vi "utility_panel.vi"() -> ()   [LabVIEW 2012]
doc: "This VI is to serve as (1) an example of how one might incorporate the many features of the stepper motor control API into their own application and (2) allows the user to take control of their hardware for demonstration and or troubleshooting purposes. Tips and descriptions have been applied to each control on the interface. Click the HELP button to see more detailed descriptions of each control and their function.\n\nProduced By:\n\nChristopher Lemieux\nKod Integrations, LLC\n4835 Marianne Drive\nMount Airy, MD 21771\nhttp://www.kodintegrations.com\nemail: clemieux@kodintegrations.com\nphone: (240) 687-1288"
uses:
  utilities/getters/controls/status_states.ctl
  support/controls/utility_actions.ctl
  main_functions/commands.ctl
  support/controls/digital_output_items.ctl
  support/controls/polarity_item_group.ctl
  support/controls/polarity_items.ctl
  support/controls/errors_actions.ctl
panel:
  in  "help":bool
  out "Current State (display)":T1(ring)=enum."CONST"
  out "Current Position (display)":i32=100 min=1 max=5000
  out "date":string
  out "power_led":bool
  in  "on/off":bool
  out "dig_ins":T2
  out "status":T3=enum."CONST"
  in  "jog_to_pos":i32 caption="Jog To Value"
  in  "move_to":bool caption="Jog To..."
  in  "home_neg":bool caption="Home (-)"
  in  "home_pos":bool caption="Home (+)"
  in  "clear":bool caption="Clear Error Codes"
  in  "Tab Control":T4(tab)
  in  "move_mode":enum32{"Abs:", "Inc:"}(radio)
  in  "position_val_set":bool
  out "position_val_actual":i32=100 min=1 max=5000
  in  "position_val_desired":i32
  in  "zero":bool
  in  "demo_start":bool
  in  "pos_3":i32
  in  "pos_2":i32
  in  "pos_1":i32
  in  "accel_set":bool
  out "accel_act":i32=100 min=1 max=5000
  in  "accel":i32=100 min=10 max=1000
  in  "low_speed_set":bool
  in  "high_speed_set":bool
  out "low_speed_act":i32=100 min=100 max=490550
  out "high_speed_act":i32=1 min=1 max=400000
  in  "low_speed":i32=100 min=100 max=490550
  in  "high_speed":i32=50 min=1 max=400000 step=1
  in  "dig_outs":T5
  out "actual_amp":i32
  in  "polarities":T6
  in  "cgh_id":bool
  in  "new_id":string
  in  "run_amp_set":bool
  in  "idle_amp_set":bool
  out "running_amp_act":i32
  out "idle_amp_act":i32
  in  "running_amp":i32=50 min=50 max=2500
  in  "idle_amp":i32=50 min=50 max=2500 step=1
  out "response":string
  out "firmware_ver":string
  out "dev_id":string
  out "prod_id":string
  in  "terminate":bool
  in  "jog_neg":bool caption="Jog (-)"
  in  "jog_pos":bool caption="Jog (+)"
  in  "imm_stop":bool caption="Stop Immediately"
  in  "slow_stop":bool caption="Stop Slowly"
  in  "raw_cmd":string
  in  "write_cmd":bool
  out "error out":errorcluster
  in  "error in (no error)":errorcluster
  # "Firmware:"
  # "Prod ID:"
  # "Dev ID:"
  # "Digital Inputs"
  # "Current Position"
  # "Current State"
  # "Status:"
  # "Mode"
  # "Speed Settings (pps)"
  # "set"
  # "(actual)"
  # "High"
  # "Low"
  # "Acceleration (ms)"
  # "set"
  # "(actual)"
  # "Accel"
  # "Demonstration"
  # "Zero First?"
  # "Position (1)"
  # "Position (2)"
  # "Position (3)"
  # "Position (ticks)"
  # "set"
  # "(actual)"
  # "new"
  # "Current Settings (mA)"
  # "set"
  # "(actual)"
  # "Idle"
  # "Run"
  # "[actual at runtime]"
  # "Polarity Settings:"
  # "Device ID:"
  # "Digital Outputs:"
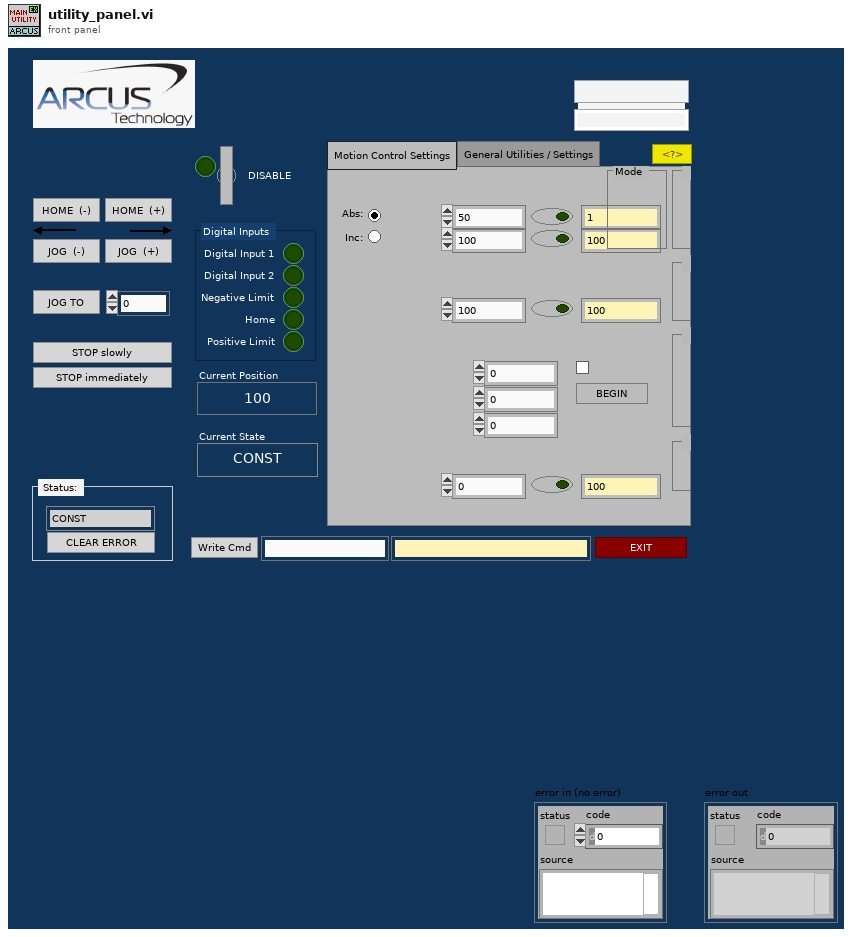
[diagram p1: front panel]
types:
  T1 = enum16{"IDLE", "CONST", "ACCEL", "DECEL", "HOME_SWITCH", "-LIMIT_SWITCH", "+LIMIT_SWITCH", "-LIMIT_ERR", "+LIMIT_ERR", "COMM_ERR"}
  T2 = cluster{"Digital Input 1":bool, "Digital Input 2":bool, "Negative Limit":bool, "Home":bool, "Positive Limit":bool}
  T3 = typedef "status_states.ctl" = enum16{"IDLE", "CONST", "ACCEL", "DECEL", "HOME_SWITCH", "-LIMIT_SWITCH", "+LIMIT_SWITCH", "-LIMIT_ERR", "+LIMIT_ERR", "COMM_ERR"}
  T4 = enum32{"Motion Control Settings", "General Utilities / Settings"}
  T5 = cluster{"Digital Output 1":bool, "Digital Output 2":bool}
  T6 = cluster{"Direction":bool, "Limit":bool, "Home":bool, "Digital Output":bool, "Digital Input":bool, "Enable Output":bool, "Jump On Error":bool}
  T7 = typedef "utility_actions.ctl" = enum16{"about", "clearError", "closeRef", "demo", "getAcceleration", "getActualCurrentVal", "getDeviceId", "getDeviceList", "getDigInputs", "getDigOutputs", "getDriverPowerStatus", "getFirmwareVer", "getHighSpeed", "getIdleCurrent", "getLowSpeed", "getMode", "getPolarity", "getPosition", "getProductId", "getRunCurrent", "getStatus", "homeMotorNeg", "homeMotorPos", "initialize", "jogConstNeg", "jogConstPos", "moveToPos", "openRef", "pause", "powerOFF", "powerON", "processEvents", "rawCmd", "setAcceleration", "setDeviceId", "setDigOutput", "setHighSpeed", "setLowSpeed", "setPolarity", "setPosition", "setRunCurrent", "setIdleCurrent", "setMode", "setTimeOuts", "stopImmediately", "stopSlowly", "storeToFlashMem", "updatePanelItems", "validateDemoPos", "validatePos", "waitUntilDone", "zeroPosition"}
  T8 = typedef "errors_actions.ctl" = enum16{"clearBuff", "closeRef", "noDeviceInfo", "noDevices", "openRef", "sendReceive", "setTimeouts", "unknown"}
  T9 = typedef "commands.ctl" = enum16{"clear error", "constant jog(-)", "constant jog(+)", "get acceleration", "get actual current", "get device id", "get digital input status", "get digial inputs status", "get dig output status", "get digital outputs status", "get firmware ver", "get high speed", "get idle current", "get low speed", "get micro step", "get motor status", "get move mode", "get polarity", "get position", "get product id", "get power status", "get run current", "get status", "home(-)", "home(+)", "move to position", "power down", "power up", "set acceleration", "set device id", "set digital output", "set digital outputs", "set high speed", "set idle current", "set low speed", "set move mode absolute", "set move mode increment", "set polarity", "set position", "set run current", "stop immediate", "stop slow", "store to memory"}
  T10 = typedef "digital_output_items.ctl" = enum16{"DIG_OUT_1", "DIG_OUT_2"}
  T11 = typedef "polarity_item_group.ctl" = cluster{"item":T12, "status":bool}
  T12 = typedef "polarity_items.ctl" = enum16{"DIRECTION", "LIMIT", "HOME", "DIG_OUT", "DIG_IN", "ENABLE_OUT", "JUMP_ERR"}
  T13 = cluster{"[0]":bool, "[1]":bool, "[2]":bool, "[3]":bool, "[4]":bool, "[5]":bool, "[6]":bool}
  T14 = typedef "digital_output_item_group.ctl" = cluster{"item":T10, "status":bool}
  T15 = typedef "digital_input_item_group.ctl" = cluster{"item":T16, "status":bool}
  T16 = typedef "digital_input_items.ctl" = enum16{"DIG_IN_1", "DIG_IN_2", "NEG_LIMIT", "HOME", "POS_LIMIT"}
  T17 = cluster{"[0]":bool, "[1]":bool, "[2]":bool, "[3]":bool, "[4]":bool}
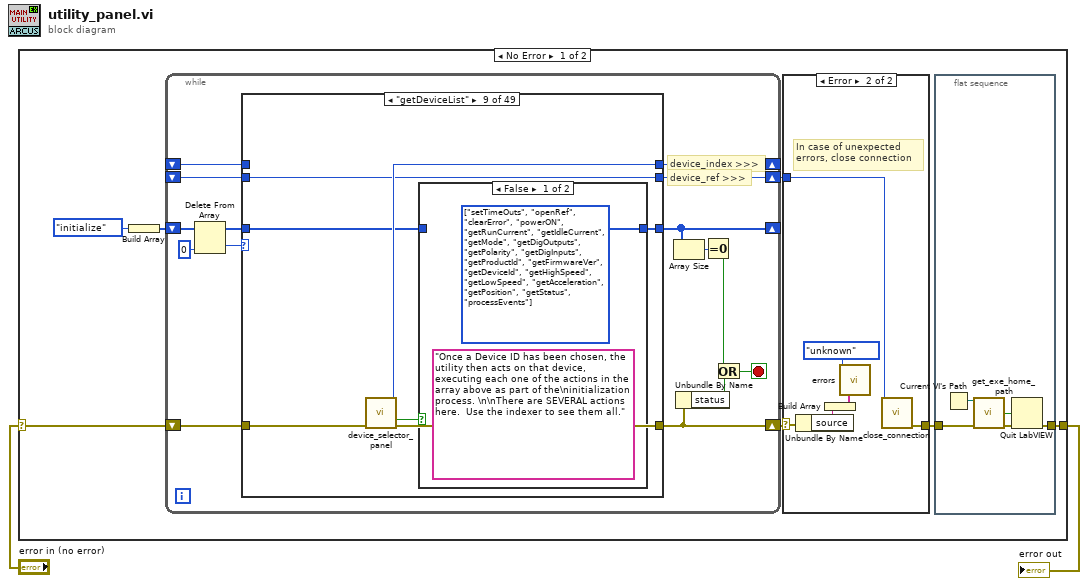
[diagram p0: block diagram]
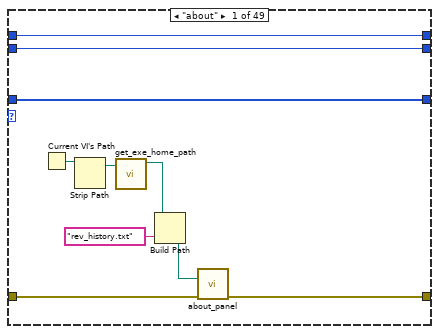
[diagram p3: hidden frame]
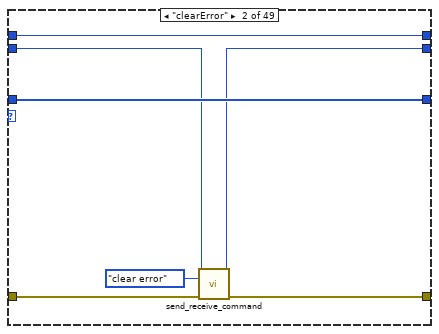
[diagram p4: hidden frame]
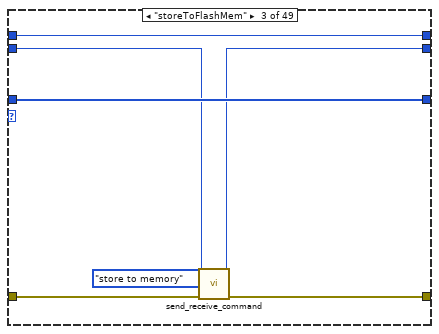
[diagram p5: hidden frame]
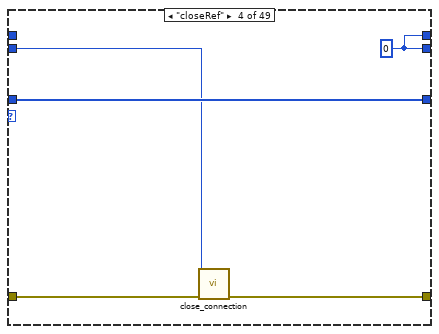
[diagram p6: hidden frame]
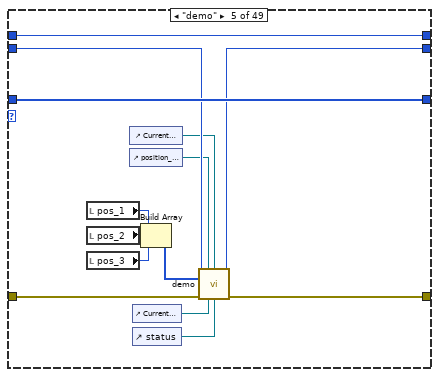
[diagram p7: hidden frame]
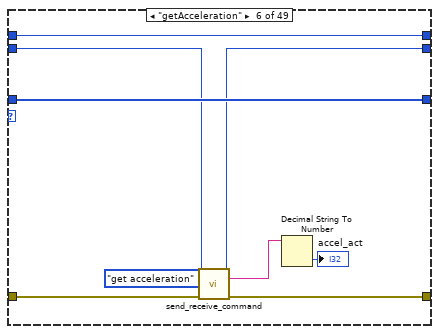
[diagram p8: hidden frame]
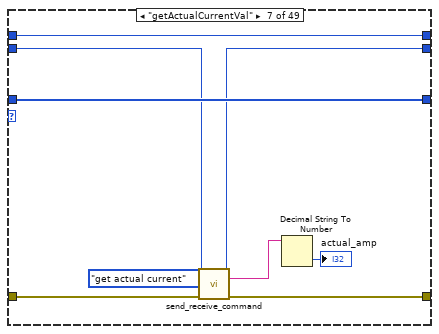
[diagram p9: hidden frame]
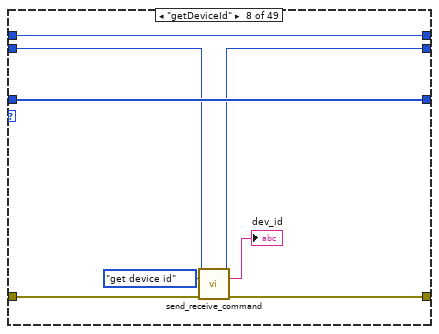
[diagram p10: hidden frame]
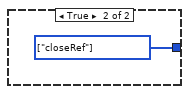
[diagram p11: hidden frame]
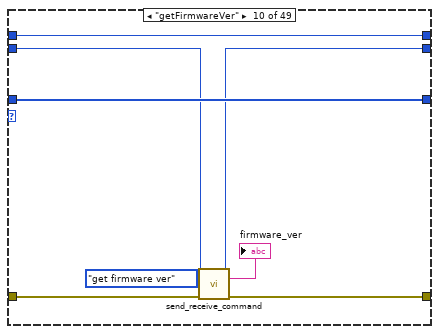
[diagram p12: hidden frame]
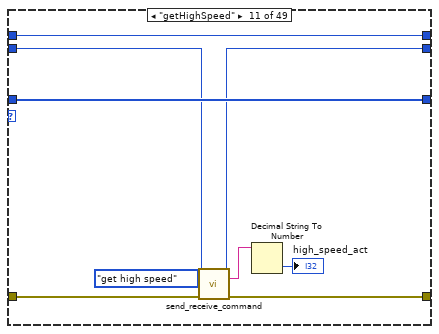
[diagram p13: hidden frame]
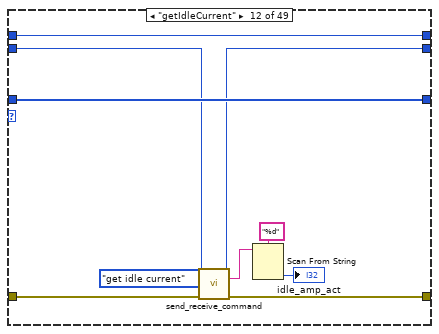
[diagram p14: hidden frame]
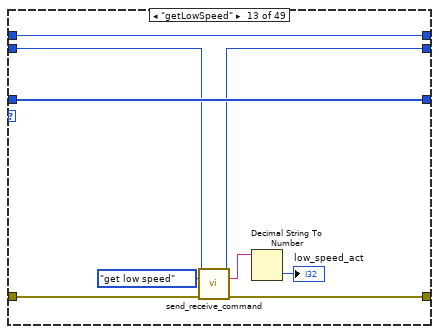
[diagram p15: hidden frame]
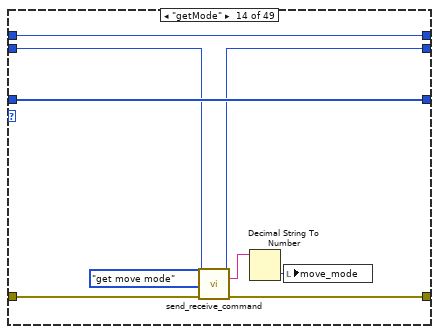
[diagram p16: hidden frame]
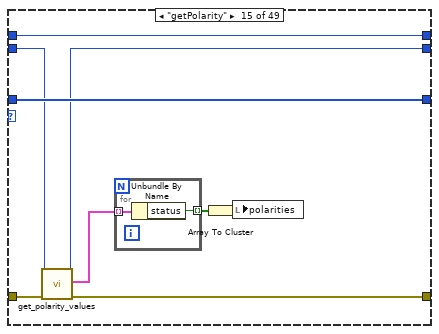
[diagram p17: hidden frame]
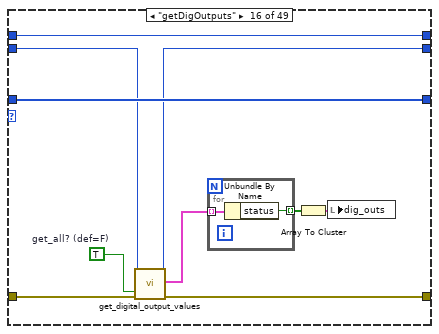
[diagram p18: hidden frame]
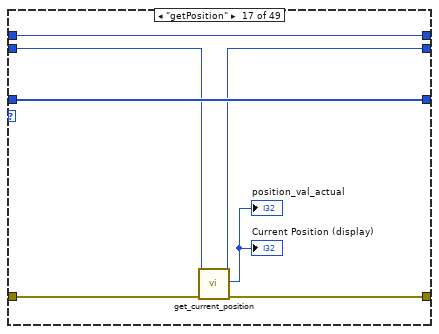
[diagram p19: hidden frame]
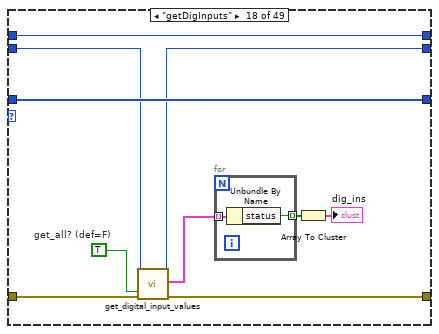
[diagram p20: hidden frame]
diagram:
  n1 = case shown="No Error" "error in (no error)" {
    selector: "error in (no error)" -> [w5 w614]
    tunnel: [w3 w614] -> w1
    frame No Error {
      n2 = Build Array(utility_actions."initialize" ("Enum")) -> (w8:T7[])
      n3 = while {
        shift-right: [w29] -> _
        shift-left: w8 -> [w34]
        shift-right: [w24] -> w7
        shift-left: w5 -> [w30]
        shift-right: [w23] -> w6
        shift-left: _ -> [w22]
        shift-right: [w21] -> _
        shift-left: _ -> [w20]
        stop <- w25 stop-if-true
        # "device_index >>>"
        # "device_ref >>>"
        n4 = Delete From Array(array=w34, index=0) -> (deleted portion=w32:T7, array with subset deleted=w31:T7[])  [unwired: 1 in]
        n5 = case shown="\"getDeviceList\"" w32 {
          tunnel: w31 -> [w44 w51 w58 w63 w73 w86 w95 w103 w105 w120 w129 w139 w148 w157 w166 w178 w187 w197 w207 w216 w223 w231 w239 _ w253 w261 w272 w278 w286 w294 w297 w399 w411 w424 w443 w455 w467 w477 w492 w502 w516 w528 w530 w544 w552 w556 w564 w590 w612]
          tunnel: [w44 w51 w58 w63 w73 w86 w95 w103 w104 w120 w129 w139 w148 w157 w166 w178 w187 w197 w207 w216 w223 w231 w239 w243 w253 w261 w271 w278 w286 w294 w298 w399 w410 w423 w442 w454 w466 w477 w491 w501 w515 w527 w530 w544 w552 w554 w560 w587 w611] -> w29
          tunnel: w30 -> [w41 w49 w56 w62 w72 w83 w93 w101 w110 w118 w127 w135 w146 w155 w164 w176 w185 w195 w205 w214 w221 w229 w237 w245 w251 w259 w270 w277 w283 w292 w301 w400 w408 w422 w440 w453 w465 w476 w490 w500 w514 w526 w534 w542 w550 w553 w561 w588 w610]
          tunnel: [w40 w48 w55 w61 w67 w82 w92 w100 w109 w117 w126 w134 w145 w154 w161 w173 w184 w194 w204 w213 w220 w225 w233 w245 w250 w258 w269 w276 w282 w291 w300 errorcluster {"status"=FALSE, "code"=0, "source"=""} w407 w414 w439 w452 w464 w475 w489 w499 w513 w525 w533 w541 w549 w553 w562 w589 w609] -> w24
          tunnel: [w42 w46 w53 w59 w70 w79 w89 w97 w107 w115 w124 w131 w143 w152 w162 w174 w182 w192 w202 w210 w218 w227 w235 w242 w248 w256 w267 w275 w280 w288 w295 w394 w405 w420 w434 w450 w462 w473 w487 w497 w511 w523 w535 w539 w547 w557 w578 w595 w607] -> w23
          tunnel: w22 -> [w42 w47 w54 w60 w71 w80 w90 w98 w107 w116 w125 w132 w144 w153 w163 w175 w183 w193 w203 w211 w219 w228 w236 _ w249 w257 w268 _ w281 w289 w295 w395 w406 w421 w438 w451 w463 w474 w488 w498 w512 w524 w535 w540 w548 w557 w578 w595 w608]
          tunnel: [w43 w50 w57 w59 w74 w85 w94 w102 w108 w119 w128 w138 w147 w156 w165 w177 w186 w196 w206 w215 w222 w230 w238 w242 w252 w260 w273 w274 w285 w293 w296 w396 w412 w425 w444 w456 w468 w478 w493 w503 w517 w529 w536 w543 w551 w558 w579 w596 w613] -> w21
          tunnel: w20 -> [w43 w50 w57 _ w74 w85 w94 w102 _ w119 w128 w138 w147 w156 w165 w177 w186 w196 w206 w215 w222 w230 w238 _ w252 w260 w273 w274 w285 w293 w296 w396 w412 w425 w444 w456 w468 w478 w493 w503 w517 w529 w536 w543 w551 w558 w579 w596 w613]
          frame "about" {
            n6 = Current VI's Path() -> (path=w37:path)
            n7 = Strip Path(path=w37) -> (stripped path=w36:path)  [unwired: 1 out]
            n8 = call "get_exe_home_path.vi"("home_path"=w36) -> ("actual_home_path"=w35:path)  [unwired: 6 in, 1 out]
            n9 = Build Path(base path=w35, name or relative path="rev_history.txt") -> (appended path=w38:path)
            n10 = call "about_panel.vi"("rev_history_filepath"=w38, "error in (no error)"=w41) -> ("error out"=w40:errorcluster)  [unwired: 13 in]
          }
          frame "clearError" {
            n11 = call "send_receive_command.vi"("reference (in)"=w47, "command"=commands."clear error" ("commands"), "error in (no error)"=w49) -> ("reference (dup)"=w46:i32, "error out"=w48:errorcluster)  [unwired: 8 in, 3 out]
          }
          frame "storeToFlashMem" {
            n12 = call "send_receive_command.vi"("reference (in)"=w54, "command"=commands."store to memory" ("commands"), "error in (no error)"=w56) -> ("reference (dup)"=w53:i32, "error out"=w55:errorcluster)  [unwired: 8 in, 3 out]
          }
          frame "closeRef" {
            w59 = 0 ("reference (out)")
            n13 = call "close_connection.vi"("reference"=w60, "error in (no error)"=w62) -> ("error out"=w61:errorcluster)  [unwired: 13 in]
          }
          frame "demo" {
            n14 = local read "pos_1"() -> (w76:i32)
            n15 = local read "pos_2"() -> (w75:i32)
            n16 = local read "pos_3"() -> (w77:i32)
            n17 = control-ref of="Current Position (display)"() -> (w66:refnum<vi>)
            n18 = control-ref of="position_val_actual"() -> (w69:refnum<vi>)
            n19 = control-ref of="Current State (display)"() -> (w65:refnum<vi>)
            n20 = control-ref of="status"() -> (w64:refnum<vi>)
            n21 = Build Array(w76, w75, w77) -> (w68:i32[])
            n22 = call "demo.vi"("reference (in)"=w71, "position ref"=w69, "position (large) ref"=w66, "positions"=w68, "error in (no error)"=w72, "Current State (display)"=w65, "status"=w64) -> ("reference (out)"=w70:i32, "error out"=w67:errorcluster)  [unwired: 7 in]
          }
          frame "getAcceleration" {
            n23 = call "send_receive_command.vi"("reference (in)"=w80, "command"=commands."get acceleration" ("commands"), "error in (no error)"=w83) -> ("reference (dup)"=w79:i32, "read_string"=w78:string, "error out"=w82:errorcluster)  [unwired: 8 in, 2 out]
            n24 = Decimal String To Number(string=w78) -> (number=→"accel_act":i32)  [unwired: 2 in, 1 out]
          }
          frame "getActualCurrentVal" {
            n25 = call "send_receive_command.vi"("reference (in)"=w90, "command"=commands."get actual current" ("commands"), "error in (no error)"=w93) -> ("reference (dup)"=w89:i32, "read_string"=w88:string, "error out"=w92:errorcluster)  [unwired: 8 in, 2 out]
            n26 = Decimal String To Number(string=w88) -> (number=→"actual_amp":i32)  [unwired: 2 in, 1 out]
          }
          frame "getDeviceId" {
            n27 = call "send_receive_command.vi"("reference (in)"=w98, "command"=commands."get device id" ("commands"), "error in (no error)"=w101) -> ("reference (dup)"=w97:i32, "read_string"=→"dev_id":string, "error out"=w100:errorcluster)  [unwired: 8 in, 2 out]
          }
          frame "getDeviceList" {
            n28 = call "device_selector_panel.vi"("error in (no error)"=w110) -> ("index"=w108:i32, "cancel?"=w106:bool, "error out"=w109:errorcluster)  [unwired: 10 in, 2 out]
            n29 = case shown="False" w106 {
              tunnel: w105 -> [_ _]
              tunnel: [w111 w112] -> w104
              frame False {
                (unwired) "Once a Device ID has been chosen, the utility then acts on that device, executing each one of the actions in the array above as part of the\ninitialization process. \n\nThere are SEVERAL actions here.  Use the indexer to see them all."
                w111 = T7[] [enum."setTimeOuts", enum."openRef", enum."clearError", enum."powerON", enum."getRunCurrent", enum."getIdleCurrent", enum."getMode", enum."getDigOutputs", enum."getPolarity", enum."getDigInputs", enum."getProductId", enum."getFirmwareVer", enum."getDeviceId", enum."getHighSpeed", enum."getLowSpeed", enum."getAcceleration", enum."getPosition", enum."getStatus", enum."processEvents"] items=["about", "clearError", "closeRef", "demo", "getAcceleration", "getActualCurrentVal", "getDeviceId", "getDeviceList", "getDigInputs", "getDigOutputs", "getDriverPowerStatus", "getFirmwareVer", "getHighSpeed", "getIdleCurrent", "getLowSpeed", "getMode", "getPolarity", "getPosition", "getProductId", "getRunCurrent", "getStatus", "homeMotorNeg", "homeMotorPos", "initialize", "jogConstNeg", "jogConstPos", "moveToPos", "openRef", "pause", "powerOFF", "powerON", "processEvents", "rawCmd", "setAcceleration", "setDeviceId", "setDigOutput", "setHighSpeed", "setLowSpeed", "setPolarity", "setPosition", "setRunCurrent", "setIdleCurrent", "setMode", "setTimeOuts", "stopImmediately", "stopSlowly", "storeToFlashMem", "updatePanelItems", "validateDemoPos", "validatePos", "waitUntilDone", "zeroPosition"] ("actions")
              }
              frame True {
                w112 = T7[] [enum."closeRef"] items=["about", "clearError", "closeRef", "demo", "getAcceleration", "getActualCurrentVal", "getDeviceId", "getDeviceList", "getDigInputs", "getDigOutputs", "getDriverPowerStatus", "getFirmwareVer", "getHighSpeed", "getIdleCurrent", "getLowSpeed", "getMode", "getPolarity", "getPosition", "getProductId", "getRunCurrent", "getStatus", "homeMotorNeg", "homeMotorPos", "initialize", "jogConstNeg", "jogConstPos", "moveToPos", "openRef", "pause", "powerOFF", "powerON", "processEvents", "rawCmd", "setAcceleration", "setDeviceId", "setDigOutput", "setHighSpeed", "setLowSpeed", "setPolarity", "setPosition", "setRunCurrent", "setIdleCurrent", "setMode", "setTimeOuts", "stopImmediately", "stopSlowly", "storeToFlashMem", "updatePanelItems", "validateDemoPos", "validatePos", "waitUntilDone", "zeroPosition"] ("actions")
              }
            }
          }
          frame "getFirmwareVer" {
            n30 = call "send_receive_command.vi"("reference (in)"=w116, "command"=commands."get firmware ver" ("commands"), "error in (no error)"=w118) -> ("reference (dup)"=w115:i32, "read_string"=→"firmware_ver":string, "error out"=w117:errorcluster)  [unwired: 8 in, 2 out]
          }
          frame "getHighSpeed" {
            n31 = call "send_receive_command.vi"("reference (in)"=w125, "command"=commands."get high speed" ("commands"), "error in (no error)"=w127) -> ("reference (dup)"=w124:i32, "read_string"=w121:string, "error out"=w126:errorcluster)  [unwired: 8 in, 2 out]
            n32 = Decimal String To Number(string=w121) -> (number=→"high_speed_act":i32)  [unwired: 2 in, 1 out]
          }
          frame "getIdleCurrent" {
            n33 = call "send_receive_command.vi"("reference (in)"=w132, "command"=commands."get idle current" ("commands"), "error in (no error)"=w135) -> ("reference (dup)"=w131:i32, "read_string"=w130:string, "error out"=w134:errorcluster)  [unwired: 8 in, 2 out]
            n34 = Scan From String(format string="%d", input string=w130) -> (output 1=→"idle_amp_act":i32)  [unwired: 3 in, 3 out]
          }
          frame "getLowSpeed" {
            n35 = call "send_receive_command.vi"("reference (in)"=w144, "command"=commands."get low speed" ("commands"), "error in (no error)"=w146) -> ("reference (dup)"=w143:i32, "read_string"=w140:string, "error out"=w145:errorcluster)  [unwired: 8 in, 2 out]
            n36 = Decimal String To Number(string=w140) -> (number=→"low_speed_act":i32)  [unwired: 2 in, 1 out]
          }
          frame "getMode" {
            n37 = call "send_receive_command.vi"("reference (in)"=w153, "command"=commands."get move mode" ("commands"), "error in (no error)"=w155) -> ("reference (dup)"=w152:i32, "read_string"=w150:string, "error out"=w154:errorcluster)  [unwired: 8 in, 2 out]
            n38 = Decimal String To Number(string=w150) -> (number=w149:i32)  [unwired: 2 in, 1 out]
            n39 = local write "move_mode"(w149) -> ()
          }
          frame "getPolarity" {
            n40 = call "get_polarity_values.vi"("reference (in)"=w163, "error in (no error)"=w164) -> ("reference (dup)"=w162:i32, "polarity_items"=w160:T11[], "error out"=w161:errorcluster)  [unwired: 14 in, 1 out]
            n41 = for {
              tunnel: w160 -> [w168] mode=indexing
              tunnel: [w167] -> w159 mode=indexing
              n42 = Unbundle By Name(w168) -> ("status"=w167:bool)
            }
            n43 = Array To Cluster(array=w159) -> (cluster=w158:T13)
            n44 = local write "polarities"(w158) -> ()
          }
          frame "getDigOutputs" {
            w169 = TRUE  # get_all? (def=F)
            n45 = call "get_digital_output_values.vi"("reference (in)"=w175, "get_all? (def=F)"=w169, "error in (no error)"=w176) -> ("reference (dup)"=w174:i32, "do_items"=w172:T14[], "error out"=w173:errorcluster)  [unwired: 12 in, 2 out]
            n46 = for {
              tunnel: w172 -> [w180] mode=indexing
              tunnel: [w179] -> w171 mode=indexing
              n47 = Unbundle By Name(w180) -> ("status"=w179:bool)
            }
            n48 = Array To Cluster(array=w171) -> (cluster=w170:cluster{"[0]":bool, "[1]":bool})
            n49 = local write "dig_outs"(w170) -> ()
          }
          frame "getPosition" {
            n50 = call "get_current_position.vi"("reference (in)"=w183, "error in (no error)"=w185) -> ("reference (dup)"=w182:i32, "current_position (units)"=→"position_val_actual" →"Current Position (display)":i32, "error out"=w184:errorcluster)  [unwired: 15 in]
          }
          frame "getDigInputs" {
            w188 = TRUE  # get_all? (def=F)
            n51 = call "get_digital_input_values.vi"("reference (in)"=w193, "get_all? (def=F)"=w188, "error in (no error)"=w195) -> ("reference (dup)"=w192:i32, "di_items"=w191:T15[], "error out"=w194:errorcluster)  [unwired: 12 in, 2 out]
            n52 = for {
              tunnel: w191 -> [w199] mode=indexing
              tunnel: [w198] -> w190 mode=indexing
              n53 = Unbundle By Name(w199) -> ("status"=w198:bool)
            }
            n54 = Array To Cluster(array=w190) -> (cluster=→"dig_ins":T17)
          }
          frame "getProductId" {
            n55 = call "send_receive_command.vi"("reference (in)"=w203, "command"=commands."get product id" ("commands"), "error in (no error)"=w205) -> ("reference (dup)"=w202:i32, "read_string"=→"prod_id":string, "error out"=w204:errorcluster)  [unwired: 8 in, 2 out]
          }
          frame "getRunCurrent" {
            n56 = call "send_receive_command.vi"("reference (in)"=w211, "command"=commands."get run current" ("commands"), "error in (no error)"=w214) -> ("reference (dup)"=w210:i32, "read_string"=w209:string, "error out"=w213:errorcluster)  [unwired: 8 in, 2 out]
            n57 = Decimal String To Number(string=w209) -> (number=→"running_amp_act":i32)  [unwired: 2 in, 1 out]
          }
          frame "getStatus" {
            n58 = call "get_status.vi"("reference (in)"=w219, "error in (no error)"=w221) -> ("reference (dup)"=w218:i32, "motion_state"=→"status" →"Current State (display)":T3, "error out"=w220:errorcluster)  [unwired: 13 in, 2 out]
          }
          frame "homeMotorNeg" {
            w224 = u8 2 ("Disabled")
            n59 = call "send_receive_command.vi"("reference (in)"=w228, "command"=commands."home(-)" ("commands"), "error in (no error)"=w229) -> ("reference (dup)"=w227:i32, "error out"=w225:errorcluster)  [unwired: 8 in, 3 out]
            n60 = property on="home_neg" class="Bool"("Disabled"=w224) -> ()  [unwired: 2 in, 2 out]
            n61 = property on="home_pos" class="Bool"("Disabled"=w224) -> ()  [unwired: 2 in, 2 out]
            n62 = property on="move_to" class="Bool"("Disabled"=w224) -> ()  [unwired: 2 in, 2 out]
            n63 = property on="jog_pos" class="Bool"("Disabled"=w224) -> ()  [unwired: 2 in, 2 out]
            n64 = property on="jog_neg" class="Bool"("Disabled"=w224) -> ()  [unwired: 2 in, 2 out]
          }
          frame "homeMotorPos" {
            w232 = u8 2 ("Disabled")
            n65 = call "send_receive_command.vi"("reference (in)"=w236, "command"=commands."home(+)" ("commands"), "error in (no error)"=w237) -> ("reference (dup)"=w235:i32, "error out"=w233:errorcluster)  [unwired: 8 in, 3 out]
            n66 = property on="home_neg" class="Bool"("Disabled"=w232) -> ()  [unwired: 2 in, 2 out]
            n67 = property on="home_pos" class="Bool"("Disabled"=w232) -> ()  [unwired: 2 in, 2 out]
            n68 = property on="move_to" class="Bool"("Disabled"=w232) -> ()  [unwired: 2 in, 2 out]
            n69 = property on="jog_pos" class="Bool"("Disabled"=w232) -> ()  [unwired: 2 in, 2 out]
            n70 = property on="jog_neg" class="Bool"("Disabled"=w232) -> ()  [unwired: 2 in, 2 out]
          }
          frame "initialize", Default {
            w240 = u8 0 ("Disabled")
            w243 = T7[] [enum."getDeviceList"] items=["about", "clearError", "closeRef", "demo", "getAcceleration", "getActualCurrentVal", "getDeviceId", "getDeviceList", "getDigInputs", "getDigOutputs", "getDriverPowerStatus", "getFirmwareVer", "getHighSpeed", "getIdleCurrent", "getLowSpeed", "getMode", "getPolarity", "getPosition", "getProductId", "getRunCurrent", "getStatus", "homeMotorNeg", "homeMotorPos", "initialize", "jogConstNeg", "jogConstPos", "moveToPos", "openRef", "pause", "powerOFF", "powerON", "processEvents", "rawCmd", "setAcceleration", "setDeviceId", "setDigOutput", "setHighSpeed", "setLowSpeed", "setPolarity", "setPosition", "setRunCurrent", "setIdleCurrent", "setMode", "setTimeOuts", "stopImmediately", "stopSlowly", "storeToFlashMem", "updatePanelItems", "validateDemoPos", "validatePos", "waitUntilDone", "zeroPosition"] ("actions")
            w242 = 0 ("index")
            w241 = ""
            w244 = FALSE
            n71 = local write "raw_cmd"(w241) -> ()
            n72 = local write "on/off"(w244) -> ()
            n73 = local write "power_led"(w244) -> ()
            n74 = local write "new_id"(w241) -> ()
            n75 = local write "response"(w241) -> ()
            n76 = property on="home_neg" class="Bool"("Disabled"=w240) -> ()  [unwired: 2 in, 2 out]
            n77 = property on="home_pos" class="Bool"("Disabled"=w240) -> ()  [unwired: 2 in, 2 out]
            n78 = property on="move_to" class="Bool"("Disabled"=w240) -> ()  [unwired: 2 in, 2 out]
            n79 = property on="jog_pos" class="Bool"("Disabled"=w240) -> ()  [unwired: 2 in, 2 out]
            n80 = property on="jog_neg" class="Bool"("Disabled"=w240) -> ()  [unwired: 2 in, 2 out]
          }
          frame "jogConstNeg" {
            w246 = u8 2 ("Disabled")
            n81 = call "send_receive_command.vi"("reference (in)"=w249, "command"=commands."constant jog(-)" ("commands"), "error in (no error)"=w251) -> ("reference (dup)"=w248:i32, "error out"=w250:errorcluster)  [unwired: 8 in, 3 out]
            n82 = property on="home_neg" class="Bool"("Disabled"=w246) -> ()  [unwired: 2 in, 2 out]
            n83 = property on="home_pos" class="Bool"("Disabled"=w246) -> ()  [unwired: 2 in, 2 out]
            n84 = property on="move_to" class="Bool"("Disabled"=w246) -> ()  [unwired: 2 in, 2 out]
            n85 = property on="jog_pos" class="Bool"("Disabled"=w246) -> ()  [unwired: 2 in, 2 out]
            n86 = property on="jog_neg" class="Bool"("Disabled"=w246) -> ()  [unwired: 2 in, 2 out]
          }
          frame "jogConstPos" {
            w254 = u8 2 ("Disabled")
            n87 = call "send_receive_command.vi"("reference (in)"=w257, "command"=commands."constant jog(+)" ("commands"), "error in (no error)"=w259) -> ("reference (dup)"=w256:i32, "error out"=w258:errorcluster)  [unwired: 8 in, 3 out]
            n88 = property on="home_neg" class="Bool"("Disabled"=w254) -> ()  [unwired: 2 in, 2 out]
            n89 = property on="home_pos" class="Bool"("Disabled"=w254) -> ()  [unwired: 2 in, 2 out]
            n90 = property on="move_to" class="Bool"("Disabled"=w254) -> ()  [unwired: 2 in, 2 out]
            n91 = property on="jog_pos" class="Bool"("Disabled"=w254) -> ()  [unwired: 2 in, 2 out]
            n92 = property on="jog_neg" class="Bool"("Disabled"=w254) -> ()  [unwired: 2 in, 2 out]
          }
          frame "moveToPos" {
            n93 = local read "jog_to_pos"() -> (w264:i32)
            n94 = Number To Decimal String(number=w264) -> (decimal integer string=w263:string)  [unwired: 1 in]
            n95 = Build Array(w263) -> (w266:string[])
            n96 = call "send_receive_command.vi"("reference (in)"=w268, "command"=commands."move to position" ("commands"), "params (opt)"=w266, "error in (no error)"=w270) -> ("reference (dup)"=w267:i32, "error out"=w269:errorcluster)  [unwired: 7 in, 3 out]
            n97 = Build Array (concatenate)(utility_actions."getPosition" ("Enum"), w272) -> (w271:T7[])
          }
          frame "openRef" {
            n98 = call "create_connection.vi"("device_index (def=0)"=w274, "error in (no error)"=w277) -> ("reference"=w275:i32, "error out"=w276:errorcluster)  [unwired: 12 in]
          }
          frame "powerOFF" {
            w279 = FALSE
            w284 = FALSE  # state (def=OFF)
            # "in the event this \ncase is triggered by\nsomething other \nthan the toggle"
            n99 = call "set_enable_disable_state.vi"("reference (in)"=w281, "state (def=OFF)"=w284, "error in (no error)"=w283) -> ("reference (dup)"=w280:i32, "error out"=w282:errorcluster)  [unwired: 14 in, 1 out]
            n100 = local write "power_led"(w279) -> ()
            n101 = local write "on/off"(w279) -> ()
          }
          frame "powerON" {
            w287 = TRUE
            w290 = TRUE  # state (def=OFF)
            # "in the event this \ncase is triggered by\nsomething other \nthan the toggle"
            n102 = call "set_enable_disable_state.vi"("reference (in)"=w289, "state (def=OFF)"=w290, "error in (no error)"=w292) -> ("reference (dup)"=w288:i32, "error out"=w291:errorcluster)  [unwired: 14 in, 1 out]
            n103 = local write "power_led"(w287) -> ()
            n104 = local write "on/off"(w287) -> ()
          }
          frame "processEvents" {
            n105 = event shown="[10] \"cgh_id\": Value Change" {
              selector: _ -> [_ _ _ _ _ _ _ _ _ _ _ _ _ _ _ _ _ _ _ _ _ _ _ _ _]
              dyn-events: _ -> [_ _ _ _ _ _ _ _ _ _ _ _ _ _ _ _ _ _ _ _ _ _ _ _ _]
              timeout: 20 -> [_ _ _ _ _ _ _ _ _ _ _ _ _ _ _ _ _ _ _ _ _ _ _ _ _]
              tunnel: [w305 w307 w309 w311 w313 w315 w317 w320 w324 w326 w335 w339 w341 w343 w345 w347 w349 w351 w354 w358 w359 w384 w388 w390 w392] -> w300
              tunnel: w301 -> [w305 w307 w309 w311 w313 w315 w317 w320 w324 w326 w335 w339 w341 w343 w345 w347 w349 w351 w354 w358 w359 w384 w388 w390 w392]
              tunnel: [w304 w306 w308 w310 w312 w314 w316 w319 w323 w325 w334 w338 w340 w342 w344 w346 w348 w350 w353 w357 w360 w383 w387 w389 w391] -> w298
              tunnel: w297 -> [_ _ _ _ _ _ _ _ _ _ _ _ _ _ _ _ _ _ _ _ _ _ _ _ _]
              event Timeout {
                w304 = T7[] [enum."updatePanelItems", enum."getDigInputs", enum."getPosition", enum."getStatus", enum."getActualCurrentVal", enum."processEvents"] items=["about", "clearError", "closeRef", "demo", "getAcceleration", "getActualCurrentVal", "getDeviceId", "getDeviceList", "getDigInputs", "getDigOutputs", "getDriverPowerStatus", "getFirmwareVer", "getHighSpeed", "getIdleCurrent", "getLowSpeed", "getMode", "getPolarity", "getPosition", "getProductId", "getRunCurrent", "getStatus", "homeMotorNeg", "homeMotorPos", "initialize", "jogConstNeg", "jogConstPos", "moveToPos", "openRef", "pause", "powerOFF", "powerON", "processEvents", "rawCmd", "setAcceleration", "setDeviceId", "setDigOutput", "setHighSpeed", "setLowSpeed", "setPolarity", "setPosition", "setRunCurrent", "setIdleCurrent", "setMode", "setTimeOuts", "stopImmediately", "stopSlowly", "storeToFlashMem", "updatePanelItems", "validateDemoPos", "validatePos", "waitUntilDone", "zeroPosition"] ("actions")
                n106 = event-data() -> ()  [unwired: 1 in, 2 out]
                n107 = Format Date/Time String(time format string (%c)="%B %d, %Y - %H:%M:%S") -> (date/time string=→"date":string)  [unwired: 2 in]
              }
              event "write_cmd": Value Change {
                w306 = T7[] [enum."rawCmd", enum."processEvents"] items=["about", "clearError", "closeRef", "demo", "getAcceleration", "getActualCurrentVal", "getDeviceId", "getDeviceList", "getDigInputs", "getDigOutputs", "getDriverPowerStatus", "getFirmwareVer", "getHighSpeed", "getIdleCurrent", "getLowSpeed", "getMode", "getPolarity", "getPosition", "getProductId", "getRunCurrent", "getStatus", "homeMotorNeg", "homeMotorPos", "initialize", "jogConstNeg", "jogConstPos", "moveToPos", "openRef", "pause", "powerOFF", "powerON", "processEvents", "rawCmd", "setAcceleration", "setDeviceId", "setDigOutput", "setHighSpeed", "setLowSpeed", "setPolarity", "setPosition", "setRunCurrent", "setIdleCurrent", "setMode", "setTimeOuts", "stopImmediately", "stopSlowly", "storeToFlashMem", "updatePanelItems", "validateDemoPos", "validatePos", "waitUntilDone", "zeroPosition"] ("actions")
                n108 = event-data() -> ()  [unwired: 1 in, 6 out]
              }
              event "slow_stop": Value Change {
                w308 = T7[] [enum."stopSlowly", enum."processEvents"] items=["about", "clearError", "closeRef", "demo", "getAcceleration", "getActualCurrentVal", "getDeviceId", "getDeviceList", "getDigInputs", "getDigOutputs", "getDriverPowerStatus", "getFirmwareVer", "getHighSpeed", "getIdleCurrent", "getLowSpeed", "getMode", "getPolarity", "getPosition", "getProductId", "getRunCurrent", "getStatus", "homeMotorNeg", "homeMotorPos", "initialize", "jogConstNeg", "jogConstPos", "moveToPos", "openRef", "pause", "powerOFF", "powerON", "processEvents", "rawCmd", "setAcceleration", "setDeviceId", "setDigOutput", "setHighSpeed", "setLowSpeed", "setPolarity", "setPosition", "setRunCurrent", "setIdleCurrent", "setMode", "setTimeOuts", "stopImmediately", "stopSlowly", "storeToFlashMem", "updatePanelItems", "validateDemoPos", "validatePos", "waitUntilDone", "zeroPosition"] ("actions")
                n109 = event-data() -> ()  [unwired: 1 in, 6 out]
              }
              event "imm_stop": Value Change {
                w310 = T7[] [enum."stopImmediately", enum."processEvents"] items=["about", "clearError", "closeRef", "demo", "getAcceleration", "getActualCurrentVal", "getDeviceId", "getDeviceList", "getDigInputs", "getDigOutputs", "getDriverPowerStatus", "getFirmwareVer", "getHighSpeed", "getIdleCurrent", "getLowSpeed", "getMode", "getPolarity", "getPosition", "getProductId", "getRunCurrent", "getStatus", "homeMotorNeg", "homeMotorPos", "initialize", "jogConstNeg", "jogConstPos", "moveToPos", "openRef", "pause", "powerOFF", "powerON", "processEvents", "rawCmd", "setAcceleration", "setDeviceId", "setDigOutput", "setHighSpeed", "setLowSpeed", "setPolarity", "setPosition", "setRunCurrent", "setIdleCurrent", "setMode", "setTimeOuts", "stopImmediately", "stopSlowly", "storeToFlashMem", "updatePanelItems", "validateDemoPos", "validatePos", "waitUntilDone", "zeroPosition"] ("actions")
                n110 = event-data() -> ()  [unwired: 1 in, 6 out]
              }
              event "jog_pos": Value Change {
                w312 = T7[] [enum."jogConstPos", enum."processEvents"] items=["about", "clearError", "closeRef", "demo", "getAcceleration", "getActualCurrentVal", "getDeviceId", "getDeviceList", "getDigInputs", "getDigOutputs", "getDriverPowerStatus", "getFirmwareVer", "getHighSpeed", "getIdleCurrent", "getLowSpeed", "getMode", "getPolarity", "getPosition", "getProductId", "getRunCurrent", "getStatus", "homeMotorNeg", "homeMotorPos", "initialize", "jogConstNeg", "jogConstPos", "moveToPos", "openRef", "pause", "powerOFF", "powerON", "processEvents", "rawCmd", "setAcceleration", "setDeviceId", "setDigOutput", "setHighSpeed", "setLowSpeed", "setPolarity", "setPosition", "setRunCurrent", "setIdleCurrent", "setMode", "setTimeOuts", "stopImmediately", "stopSlowly", "storeToFlashMem", "updatePanelItems", "validateDemoPos", "validatePos", "waitUntilDone", "zeroPosition"] ("actions")
                n111 = event-data() -> ()  [unwired: 1 in, 6 out]
              }
              event "jog_neg": Value Change {
                w314 = T7[] [enum."jogConstNeg", enum."processEvents"] items=["about", "clearError", "closeRef", "demo", "getAcceleration", "getActualCurrentVal", "getDeviceId", "getDeviceList", "getDigInputs", "getDigOutputs", "getDriverPowerStatus", "getFirmwareVer", "getHighSpeed", "getIdleCurrent", "getLowSpeed", "getMode", "getPolarity", "getPosition", "getProductId", "getRunCurrent", "getStatus", "homeMotorNeg", "homeMotorPos", "initialize", "jogConstNeg", "jogConstPos", "moveToPos", "openRef", "pause", "powerOFF", "powerON", "processEvents", "rawCmd", "setAcceleration", "setDeviceId", "setDigOutput", "setHighSpeed", "setLowSpeed", "setPolarity", "setPosition", "setRunCurrent", "setIdleCurrent", "setMode", "setTimeOuts", "stopImmediately", "stopSlowly", "storeToFlashMem", "updatePanelItems", "validateDemoPos", "validatePos", "waitUntilDone", "zeroPosition"] ("actions")
                n112 = event-data() -> ()  [unwired: 1 in, 6 out]
              }
              event "terminate": Value Change {
                w316 = T7[] [enum."powerOFF", enum."closeRef"] items=["about", "clearError", "closeRef", "demo", "getAcceleration", "getActualCurrentVal", "getDeviceId", "getDeviceList", "getDigInputs", "getDigOutputs", "getDriverPowerStatus", "getFirmwareVer", "getHighSpeed", "getIdleCurrent", "getLowSpeed", "getMode", "getPolarity", "getPosition", "getProductId", "getRunCurrent", "getStatus", "homeMotorNeg", "homeMotorPos", "initialize", "jogConstNeg", "jogConstPos", "moveToPos", "openRef", "pause", "powerOFF", "powerON", "processEvents", "rawCmd", "setAcceleration", "setDeviceId", "setDigOutput", "setHighSpeed", "setLowSpeed", "setPolarity", "setPosition", "setRunCurrent", "setIdleCurrent", "setMode", "setTimeOuts", "stopImmediately", "stopSlowly", "storeToFlashMem", "updatePanelItems", "validateDemoPos", "validatePos", "waitUntilDone", "zeroPosition"] ("actions")
                n113 = event-data() -> ()  [unwired: 1 in, 6 out]
              }
              event "on/off": Value Change {
                n114 = event-data() -> ("NewVal"=w318:bool)  [unwired: 1 in, 5 out]
                "power_led" <- w318
                n115 = case shown="False" w318 {
                  tunnel: [w321 w322] -> w319
                  frame True {
                    w321 = T7[] [enum."powerON", enum."processEvents"] items=["about", "clearError", "closeRef", "demo", "getAcceleration", "getActualCurrentVal", "getDeviceId", "getDeviceList", "getDigInputs", "getDigOutputs", "getDriverPowerStatus", "getFirmwareVer", "getHighSpeed", "getIdleCurrent", "getLowSpeed", "getMode", "getPolarity", "getPosition", "getProductId", "getRunCurrent", "getStatus", "homeMotorNeg", "homeMotorPos", "initialize", "jogConstNeg", "jogConstPos", "moveToPos", "openRef", "pause", "powerOFF", "powerON", "processEvents", "rawCmd", "setAcceleration", "setDeviceId", "setDigOutput", "setHighSpeed", "setLowSpeed", "setPolarity", "setPosition", "setRunCurrent", "setIdleCurrent", "setMode", "setTimeOuts", "stopImmediately", "stopSlowly", "storeToFlashMem", "updatePanelItems", "validateDemoPos", "validatePos", "waitUntilDone", "zeroPosition"] ("actions")
                  }
                  frame False {
                    w322 = T7[] [enum."powerOFF", enum."processEvents"] items=["about", "clearError", "closeRef", "demo", "getAcceleration", "getActualCurrentVal", "getDeviceId", "getDeviceList", "getDigInputs", "getDigOutputs", "getDriverPowerStatus", "getFirmwareVer", "getHighSpeed", "getIdleCurrent", "getLowSpeed", "getMode", "getPolarity", "getPosition", "getProductId", "getRunCurrent", "getStatus", "homeMotorNeg", "homeMotorPos", "initialize", "jogConstNeg", "jogConstPos", "moveToPos", "openRef", "pause", "powerOFF", "powerON", "processEvents", "rawCmd", "setAcceleration", "setDeviceId", "setDigOutput", "setHighSpeed", "setLowSpeed", "setPolarity", "setPosition", "setRunCurrent", "setIdleCurrent", "setMode", "setTimeOuts", "stopImmediately", "stopSlowly", "storeToFlashMem", "updatePanelItems", "validateDemoPos", "validatePos", "waitUntilDone", "zeroPosition"] ("actions")
                  }
                }
              }
              event "idle_amp_set": Value Change {
                w323 = T7[] [enum."setIdleCurrent", enum."processEvents"] items=["about", "clearError", "closeRef", "demo", "getAcceleration", "getActualCurrentVal", "getDeviceId", "getDeviceList", "getDigInputs", "getDigOutputs", "getDriverPowerStatus", "getFirmwareVer", "getHighSpeed", "getIdleCurrent", "getLowSpeed", "getMode", "getPolarity", "getPosition", "getProductId", "getRunCurrent", "getStatus", "homeMotorNeg", "homeMotorPos", "initialize", "jogConstNeg", "jogConstPos", "moveToPos", "openRef", "pause", "powerOFF", "powerON", "processEvents", "rawCmd", "setAcceleration", "setDeviceId", "setDigOutput", "setHighSpeed", "setLowSpeed", "setPolarity", "setPosition", "setRunCurrent", "setIdleCurrent", "setMode", "setTimeOuts", "stopImmediately", "stopSlowly", "storeToFlashMem", "updatePanelItems", "validateDemoPos", "validatePos", "waitUntilDone", "zeroPosition"] ("actions")
                n116 = event-data() -> ()  [unwired: 1 in, 6 out]
              }
              event "run_amp_set": Value Change {
                w325 = T7[] [enum."setRunCurrent", enum."processEvents"] items=["about", "clearError", "closeRef", "demo", "getAcceleration", "getActualCurrentVal", "getDeviceId", "getDeviceList", "getDigInputs", "getDigOutputs", "getDriverPowerStatus", "getFirmwareVer", "getHighSpeed", "getIdleCurrent", "getLowSpeed", "getMode", "getPolarity", "getPosition", "getProductId", "getRunCurrent", "getStatus", "homeMotorNeg", "homeMotorPos", "initialize", "jogConstNeg", "jogConstPos", "moveToPos", "openRef", "pause", "powerOFF", "powerON", "processEvents", "rawCmd", "setAcceleration", "setDeviceId", "setDigOutput", "setHighSpeed", "setLowSpeed", "setPolarity", "setPosition", "setRunCurrent", "setIdleCurrent", "setMode", "setTimeOuts", "stopImmediately", "stopSlowly", "storeToFlashMem", "updatePanelItems", "validateDemoPos", "validatePos", "waitUntilDone", "zeroPosition"] ("actions")
                n117 = event-data() -> ()  [unwired: 1 in, 6 out]
              }
              event "cgh_id": Value Change {
                n118 = event-data() -> ()  [unwired: 1 in, 6 out]
                n119 = local read "new_id"() -> (w331:string)
                n120 = local read "dev_id"() -> (w332:string)
                n121 = Format Into String(format string="Are you sure you want to change the\nDevice ID from '%s' to '%s'?", w332, w331) -> (resulting string=w330:string)  [unwired: 2 in, 1 out]
                n122 = Two Button Dialog(message=w330, 1:"Cancel" ("T button name (\"OK\")"), 2:"Yes" ("T button name (\"OK\")")) -> (T button?=w327:bool)
                n123 = case shown="False" w327 {
                  tunnel: [w336 w337] -> w334
                  frame True {
                    w336 = T7[] [enum."setDeviceId", enum."processEvents"] items=["about", "clearError", "closeRef", "demo", "getAcceleration", "getActualCurrentVal", "getDeviceId", "getDeviceList", "getDigInputs", "getDigOutputs", "getDriverPowerStatus", "getFirmwareVer", "getHighSpeed", "getIdleCurrent", "getLowSpeed", "getMode", "getPolarity", "getPosition", "getProductId", "getRunCurrent", "getStatus", "homeMotorNeg", "homeMotorPos", "initialize", "jogConstNeg", "jogConstPos", "moveToPos", "openRef", "pause", "powerOFF", "powerON", "processEvents", "rawCmd", "setAcceleration", "setDeviceId", "setDigOutput", "setHighSpeed", "setLowSpeed", "setPolarity", "setPosition", "setRunCurrent", "setIdleCurrent", "setMode", "setTimeOuts", "stopImmediately", "stopSlowly", "storeToFlashMem", "updatePanelItems", "validateDemoPos", "validatePos", "waitUntilDone", "zeroPosition"] ("actions")
                  }
                  frame False {
                    w337 = T7[] [enum."processEvents"] items=["about", "clearError", "closeRef", "demo", "getAcceleration", "getActualCurrentVal", "getDeviceId", "getDeviceList", "getDigInputs", "getDigOutputs", "getDriverPowerStatus", "getFirmwareVer", "getHighSpeed", "getIdleCurrent", "getLowSpeed", "getMode", "getPolarity", "getPosition", "getProductId", "getRunCurrent", "getStatus", "homeMotorNeg", "homeMotorPos", "initialize", "jogConstNeg", "jogConstPos", "moveToPos", "openRef", "pause", "powerOFF", "powerON", "processEvents", "rawCmd", "setAcceleration", "setDeviceId", "setDigOutput", "setHighSpeed", "setLowSpeed", "setPolarity", "setPosition", "setRunCurrent", "setIdleCurrent", "setMode", "setTimeOuts", "stopImmediately", "stopSlowly", "storeToFlashMem", "updatePanelItems", "validateDemoPos", "validatePos", "waitUntilDone", "zeroPosition"] ("actions")
                  }
                }
              }
              event "high_speed_set": Value Change {
                w338 = T7[] [enum."setHighSpeed", enum."processEvents"] items=["about", "clearError", "closeRef", "demo", "getAcceleration", "getActualCurrentVal", "getDeviceId", "getDeviceList", "getDigInputs", "getDigOutputs", "getDriverPowerStatus", "getFirmwareVer", "getHighSpeed", "getIdleCurrent", "getLowSpeed", "getMode", "getPolarity", "getPosition", "getProductId", "getRunCurrent", "getStatus", "homeMotorNeg", "homeMotorPos", "initialize", "jogConstNeg", "jogConstPos", "moveToPos", "openRef", "pause", "powerOFF", "powerON", "processEvents", "rawCmd", "setAcceleration", "setDeviceId", "setDigOutput", "setHighSpeed", "setLowSpeed", "setPolarity", "setPosition", "setRunCurrent", "setIdleCurrent", "setMode", "setTimeOuts", "stopImmediately", "stopSlowly", "storeToFlashMem", "updatePanelItems", "validateDemoPos", "validatePos", "waitUntilDone", "zeroPosition"] ("actions")
                n124 = event-data() -> ()  [unwired: 1 in, 6 out]
              }
              event "low_speed_set": Value Change {
                w340 = T7[] [enum."setLowSpeed", enum."processEvents"] items=["about", "clearError", "closeRef", "demo", "getAcceleration", "getActualCurrentVal", "getDeviceId", "getDeviceList", "getDigInputs", "getDigOutputs", "getDriverPowerStatus", "getFirmwareVer", "getHighSpeed", "getIdleCurrent", "getLowSpeed", "getMode", "getPolarity", "getPosition", "getProductId", "getRunCurrent", "getStatus", "homeMotorNeg", "homeMotorPos", "initialize", "jogConstNeg", "jogConstPos", "moveToPos", "openRef", "pause", "powerOFF", "powerON", "processEvents", "rawCmd", "setAcceleration", "setDeviceId", "setDigOutput", "setHighSpeed", "setLowSpeed", "setPolarity", "setPosition", "setRunCurrent", "setIdleCurrent", "setMode", "setTimeOuts", "stopImmediately", "stopSlowly", "storeToFlashMem", "updatePanelItems", "validateDemoPos", "validatePos", "waitUntilDone", "zeroPosition"] ("actions")
                n125 = event-data() -> ()  [unwired: 1 in, 6 out]
              }
              event "accel_set": Value Change {
                w342 = T7[] [enum."setAcceleration", enum."processEvents"] items=["about", "clearError", "closeRef", "demo", "getAcceleration", "getActualCurrentVal", "getDeviceId", "getDeviceList", "getDigInputs", "getDigOutputs", "getDriverPowerStatus", "getFirmwareVer", "getHighSpeed", "getIdleCurrent", "getLowSpeed", "getMode", "getPolarity", "getPosition", "getProductId", "getRunCurrent", "getStatus", "homeMotorNeg", "homeMotorPos", "initialize", "jogConstNeg", "jogConstPos", "moveToPos", "openRef", "pause", "powerOFF", "powerON", "processEvents", "rawCmd", "setAcceleration", "setDeviceId", "setDigOutput", "setHighSpeed", "setLowSpeed", "setPolarity", "setPosition", "setRunCurrent", "setIdleCurrent", "setMode", "setTimeOuts", "stopImmediately", "stopSlowly", "storeToFlashMem", "updatePanelItems", "validateDemoPos", "validatePos", "waitUntilDone", "zeroPosition"] ("actions")
                n126 = event-data() -> ()  [unwired: 1 in, 6 out]
              }
              event "clear": Value Change {
                w344 = T7[] [enum."clearError", enum."processEvents"] items=["about", "clearError", "closeRef", "demo", "getAcceleration", "getActualCurrentVal", "getDeviceId", "getDeviceList", "getDigInputs", "getDigOutputs", "getDriverPowerStatus", "getFirmwareVer", "getHighSpeed", "getIdleCurrent", "getLowSpeed", "getMode", "getPolarity", "getPosition", "getProductId", "getRunCurrent", "getStatus", "homeMotorNeg", "homeMotorPos", "initialize", "jogConstNeg", "jogConstPos", "moveToPos", "openRef", "pause", "powerOFF", "powerON", "processEvents", "rawCmd", "setAcceleration", "setDeviceId", "setDigOutput", "setHighSpeed", "setLowSpeed", "setPolarity", "setPosition", "setRunCurrent", "setIdleCurrent", "setMode", "setTimeOuts", "stopImmediately", "stopSlowly", "storeToFlashMem", "updatePanelItems", "validateDemoPos", "validatePos", "waitUntilDone", "zeroPosition"] ("actions")
                n127 = event-data() -> ()  [unwired: 1 in, 6 out]
              }
              event "home_pos": Value Change {
                w346 = T7[] [enum."homeMotorPos", enum."processEvents"] items=["about", "clearError", "closeRef", "demo", "getAcceleration", "getActualCurrentVal", "getDeviceId", "getDeviceList", "getDigInputs", "getDigOutputs", "getDriverPowerStatus", "getFirmwareVer", "getHighSpeed", "getIdleCurrent", "getLowSpeed", "getMode", "getPolarity", "getPosition", "getProductId", "getRunCurrent", "getStatus", "homeMotorNeg", "homeMotorPos", "initialize", "jogConstNeg", "jogConstPos", "moveToPos", "openRef", "pause", "powerOFF", "powerON", "processEvents", "rawCmd", "setAcceleration", "setDeviceId", "setDigOutput", "setHighSpeed", "setLowSpeed", "setPolarity", "setPosition", "setRunCurrent", "setIdleCurrent", "setMode", "setTimeOuts", "stopImmediately", "stopSlowly", "storeToFlashMem", "updatePanelItems", "validateDemoPos", "validatePos", "waitUntilDone", "zeroPosition"] ("actions")
                n128 = event-data() -> ()  [unwired: 1 in, 6 out]
              }
              event "home_neg": Value Change {
                w348 = T7[] [enum."homeMotorNeg", enum."processEvents"] items=["about", "clearError", "closeRef", "demo", "getAcceleration", "getActualCurrentVal", "getDeviceId", "getDeviceList", "getDigInputs", "getDigOutputs", "getDriverPowerStatus", "getFirmwareVer", "getHighSpeed", "getIdleCurrent", "getLowSpeed", "getMode", "getPolarity", "getPosition", "getProductId", "getRunCurrent", "getStatus", "homeMotorNeg", "homeMotorPos", "initialize", "jogConstNeg", "jogConstPos", "moveToPos", "openRef", "pause", "powerOFF", "powerON", "processEvents", "rawCmd", "setAcceleration", "setDeviceId", "setDigOutput", "setHighSpeed", "setLowSpeed", "setPolarity", "setPosition", "setRunCurrent", "setIdleCurrent", "setMode", "setTimeOuts", "stopImmediately", "stopSlowly", "storeToFlashMem", "updatePanelItems", "validateDemoPos", "validatePos", "waitUntilDone", "zeroPosition"] ("actions")
                n129 = event-data() -> ()  [unwired: 1 in, 6 out]
              }
              event "position_val_set": Value Change {
                w350 = T7[] [enum."setPosition", enum."processEvents"] items=["about", "clearError", "closeRef", "demo", "getAcceleration", "getActualCurrentVal", "getDeviceId", "getDeviceList", "getDigInputs", "getDigOutputs", "getDriverPowerStatus", "getFirmwareVer", "getHighSpeed", "getIdleCurrent", "getLowSpeed", "getMode", "getPolarity", "getPosition", "getProductId", "getRunCurrent", "getStatus", "homeMotorNeg", "homeMotorPos", "initialize", "jogConstNeg", "jogConstPos", "moveToPos", "openRef", "pause", "powerOFF", "powerON", "processEvents", "rawCmd", "setAcceleration", "setDeviceId", "setDigOutput", "setHighSpeed", "setLowSpeed", "setPolarity", "setPosition", "setRunCurrent", "setIdleCurrent", "setMode", "setTimeOuts", "stopImmediately", "stopSlowly", "storeToFlashMem", "updatePanelItems", "validateDemoPos", "validatePos", "waitUntilDone", "zeroPosition"] ("actions")
                n130 = event-data() -> ()  [unwired: 1 in, 6 out]
              }
              event "demo_start": Value Change {
                n131 = event-data() -> ()  [unwired: 1 in, 6 out]
                n132 = case shown="True" "zero" {
                  tunnel: [w355 w356] -> w353
                  frame True {
                    w355 = T7[] [enum."zeroPosition", enum."demo", enum."processEvents"] items=["about", "clearError", "closeRef", "demo", "getAcceleration", "getActualCurrentVal", "getDeviceId", "getDeviceList", "getDigInputs", "getDigOutputs", "getDriverPowerStatus", "getFirmwareVer", "getHighSpeed", "getIdleCurrent", "getLowSpeed", "getMode", "getPolarity", "getPosition", "getProductId", "getRunCurrent", "getStatus", "homeMotorNeg", "homeMotorPos", "initialize", "jogConstNeg", "jogConstPos", "moveToPos", "openRef", "pause", "powerOFF", "powerON", "processEvents", "rawCmd", "setAcceleration", "setDeviceId", "setDigOutput", "setHighSpeed", "setLowSpeed", "setPolarity", "setPosition", "setRunCurrent", "setIdleCurrent", "setMode", "setTimeOuts", "stopImmediately", "stopSlowly", "storeToFlashMem", "updatePanelItems", "validateDemoPos", "validatePos", "waitUntilDone", "zeroPosition"] ("actions")
                  }
                  frame False {
                    w356 = T7[] [enum."demo", enum."processEvents"] items=["about", "clearError", "closeRef", "demo", "getAcceleration", "getActualCurrentVal", "getDeviceId", "getDeviceList", "getDigInputs", "getDigOutputs", "getDriverPowerStatus", "getFirmwareVer", "getHighSpeed", "getIdleCurrent", "getLowSpeed", "getMode", "getPolarity", "getPosition", "getProductId", "getRunCurrent", "getStatus", "homeMotorNeg", "homeMotorPos", "initialize", "jogConstNeg", "jogConstPos", "moveToPos", "openRef", "pause", "powerOFF", "powerON", "processEvents", "rawCmd", "setAcceleration", "setDeviceId", "setDigOutput", "setHighSpeed", "setLowSpeed", "setPolarity", "setPosition", "setRunCurrent", "setIdleCurrent", "setMode", "setTimeOuts", "stopImmediately", "stopSlowly", "storeToFlashMem", "updatePanelItems", "validateDemoPos", "validatePos", "waitUntilDone", "zeroPosition"] ("actions")
                  }
                }
              }
              event "move_to": Value Change {
                w357 = T7[] [enum."validatePos", enum."moveToPos", enum."processEvents"] items=["about", "clearError", "closeRef", "demo", "getAcceleration", "getActualCurrentVal", "getDeviceId", "getDeviceList", "getDigInputs", "getDigOutputs", "getDriverPowerStatus", "getFirmwareVer", "getHighSpeed", "getIdleCurrent", "getLowSpeed", "getMode", "getPolarity", "getPosition", "getProductId", "getRunCurrent", "getStatus", "homeMotorNeg", "homeMotorPos", "initialize", "jogConstNeg", "jogConstPos", "moveToPos", "openRef", "pause", "powerOFF", "powerON", "processEvents", "rawCmd", "setAcceleration", "setDeviceId", "setDigOutput", "setHighSpeed", "setLowSpeed", "setPolarity", "setPosition", "setRunCurrent", "setIdleCurrent", "setMode", "setTimeOuts", "stopImmediately", "stopSlowly", "storeToFlashMem", "updatePanelItems", "validateDemoPos", "validatePos", "waitUntilDone", "zeroPosition"] ("actions")
                n133 = event-data() -> ()  [unwired: 1 in, 6 out]
              }
              event Menu Selection (User) {
                n134 = event-data() -> ("ItemTag"=w362:string)  [unwired: 1 in, 6 out]
                n135 = To Lower Case(string=w362) -> (all lower case string=w361:string)
                n136 = case shown="\"toggle on/off\"" w361 {
                  selector: w361 -> [_ _ _ _ _ _ _ _ _ _ _ w379]
                  tunnel: [w363 w365 w366 w367 w368 w370 w371 w372 w373 w374 w376 w382] -> w360
                  frame "about" {
                    w363 = T7[] [enum."about", enum."processEvents"] items=["about", "clearError", "closeRef", "demo", "getAcceleration", "getActualCurrentVal", "getDeviceId", "getDeviceList", "getDigInputs", "getDigOutputs", "getDriverPowerStatus", "getFirmwareVer", "getHighSpeed", "getIdleCurrent", "getLowSpeed", "getMode", "getPolarity", "getPosition", "getProductId", "getRunCurrent", "getStatus", "homeMotorNeg", "homeMotorPos", "initialize", "jogConstNeg", "jogConstPos", "moveToPos", "openRef", "pause", "powerOFF", "powerON", "processEvents", "rawCmd", "setAcceleration", "setDeviceId", "setDigOutput", "setHighSpeed", "setLowSpeed", "setPolarity", "setPosition", "setRunCurrent", "setIdleCurrent", "setMode", "setTimeOuts", "stopImmediately", "stopSlowly", "storeToFlashMem", "updatePanelItems", "validateDemoPos", "validatePos", "waitUntilDone", "zeroPosition"] ("actions")
                  }
                  frame "absolute" {
                    w365 = T7[] [enum."setMode", enum."processEvents"] items=["about", "clearError", "closeRef", "demo", "getAcceleration", "getActualCurrentVal", "getDeviceId", "getDeviceList", "getDigInputs", "getDigOutputs", "getDriverPowerStatus", "getFirmwareVer", "getHighSpeed", "getIdleCurrent", "getLowSpeed", "getMode", "getPolarity", "getPosition", "getProductId", "getRunCurrent", "getStatus", "homeMotorNeg", "homeMotorPos", "initialize", "jogConstNeg", "jogConstPos", "moveToPos", "openRef", "pause", "powerOFF", "powerON", "processEvents", "rawCmd", "setAcceleration", "setDeviceId", "setDigOutput", "setHighSpeed", "setLowSpeed", "setPolarity", "setPosition", "setRunCurrent", "setIdleCurrent", "setMode", "setTimeOuts", "stopImmediately", "stopSlowly", "storeToFlashMem", "updatePanelItems", "validateDemoPos", "validatePos", "waitUntilDone", "zeroPosition"] ("actions")
                    n137 = local write "move_mode"(enum32{"Abs:", "Inc:"}."Abs:" ("move_mode")) -> ()
                  }
                  frame "exit" {
                    w366 = T7[] [enum."powerOFF", enum."closeRef"] items=["about", "clearError", "closeRef", "demo", "getAcceleration", "getActualCurrentVal", "getDeviceId", "getDeviceList", "getDigInputs", "getDigOutputs", "getDriverPowerStatus", "getFirmwareVer", "getHighSpeed", "getIdleCurrent", "getLowSpeed", "getMode", "getPolarity", "getPosition", "getProductId", "getRunCurrent", "getStatus", "homeMotorNeg", "homeMotorPos", "initialize", "jogConstNeg", "jogConstPos", "moveToPos", "openRef", "pause", "powerOFF", "powerON", "processEvents", "rawCmd", "setAcceleration", "setDeviceId", "setDigOutput", "setHighSpeed", "setLowSpeed", "setPolarity", "setPosition", "setRunCurrent", "setIdleCurrent", "setMode", "setTimeOuts", "stopImmediately", "stopSlowly", "storeToFlashMem", "updatePanelItems", "validateDemoPos", "validatePos", "waitUntilDone", "zeroPosition"] ("actions")
                  }
                  frame "home (+)" {
                    w367 = T7[] [enum."homeMotorPos", enum."processEvents"] items=["about", "clearError", "closeRef", "demo", "getAcceleration", "getActualCurrentVal", "getDeviceId", "getDeviceList", "getDigInputs", "getDigOutputs", "getDriverPowerStatus", "getFirmwareVer", "getHighSpeed", "getIdleCurrent", "getLowSpeed", "getMode", "getPolarity", "getPosition", "getProductId", "getRunCurrent", "getStatus", "homeMotorNeg", "homeMotorPos", "initialize", "jogConstNeg", "jogConstPos", "moveToPos", "openRef", "pause", "powerOFF", "powerON", "processEvents", "rawCmd", "setAcceleration", "setDeviceId", "setDigOutput", "setHighSpeed", "setLowSpeed", "setPolarity", "setPosition", "setRunCurrent", "setIdleCurrent", "setMode", "setTimeOuts", "stopImmediately", "stopSlowly", "storeToFlashMem", "updatePanelItems", "validateDemoPos", "validatePos", "waitUntilDone", "zeroPosition"] ("actions")
                  }
                  frame "home (-)" {
                    w368 = T7[] [enum."homeMotorNeg", enum."processEvents"] items=["about", "clearError", "closeRef", "demo", "getAcceleration", "getActualCurrentVal", "getDeviceId", "getDeviceList", "getDigInputs", "getDigOutputs", "getDriverPowerStatus", "getFirmwareVer", "getHighSpeed", "getIdleCurrent", "getLowSpeed", "getMode", "getPolarity", "getPosition", "getProductId", "getRunCurrent", "getStatus", "homeMotorNeg", "homeMotorPos", "initialize", "jogConstNeg", "jogConstPos", "moveToPos", "openRef", "pause", "powerOFF", "powerON", "processEvents", "rawCmd", "setAcceleration", "setDeviceId", "setDigOutput", "setHighSpeed", "setLowSpeed", "setPolarity", "setPosition", "setRunCurrent", "setIdleCurrent", "setMode", "setTimeOuts", "stopImmediately", "stopSlowly", "storeToFlashMem", "updatePanelItems", "validateDemoPos", "validatePos", "waitUntilDone", "zeroPosition"] ("actions")
                  }
                  frame "incremental" {
                    w370 = T7[] [enum."setMode", enum."processEvents"] items=["about", "clearError", "closeRef", "demo", "getAcceleration", "getActualCurrentVal", "getDeviceId", "getDeviceList", "getDigInputs", "getDigOutputs", "getDriverPowerStatus", "getFirmwareVer", "getHighSpeed", "getIdleCurrent", "getLowSpeed", "getMode", "getPolarity", "getPosition", "getProductId", "getRunCurrent", "getStatus", "homeMotorNeg", "homeMotorPos", "initialize", "jogConstNeg", "jogConstPos", "moveToPos", "openRef", "pause", "powerOFF", "powerON", "processEvents", "rawCmd", "setAcceleration", "setDeviceId", "setDigOutput", "setHighSpeed", "setLowSpeed", "setPolarity", "setPosition", "setRunCurrent", "setIdleCurrent", "setMode", "setTimeOuts", "stopImmediately", "stopSlowly", "storeToFlashMem", "updatePanelItems", "validateDemoPos", "validatePos", "waitUntilDone", "zeroPosition"] ("actions")
                    n138 = local write "move_mode"(enum32{"Abs:", "Inc:"}."Inc:" ("move_mode")) -> ()
                  }
                  frame "jog (+)" {
                    w371 = T7[] [enum."jogConstPos", enum."processEvents"] items=["about", "clearError", "closeRef", "demo", "getAcceleration", "getActualCurrentVal", "getDeviceId", "getDeviceList", "getDigInputs", "getDigOutputs", "getDriverPowerStatus", "getFirmwareVer", "getHighSpeed", "getIdleCurrent", "getLowSpeed", "getMode", "getPolarity", "getPosition", "getProductId", "getRunCurrent", "getStatus", "homeMotorNeg", "homeMotorPos", "initialize", "jogConstNeg", "jogConstPos", "moveToPos", "openRef", "pause", "powerOFF", "powerON", "processEvents", "rawCmd", "setAcceleration", "setDeviceId", "setDigOutput", "setHighSpeed", "setLowSpeed", "setPolarity", "setPosition", "setRunCurrent", "setIdleCurrent", "setMode", "setTimeOuts", "stopImmediately", "stopSlowly", "storeToFlashMem", "updatePanelItems", "validateDemoPos", "validatePos", "waitUntilDone", "zeroPosition"] ("actions")
                  }
                  frame "jog (-)" {
                    w372 = T7[] [enum."jogConstNeg", enum."processEvents"] items=["about", "clearError", "closeRef", "demo", "getAcceleration", "getActualCurrentVal", "getDeviceId", "getDeviceList", "getDigInputs", "getDigOutputs", "getDriverPowerStatus", "getFirmwareVer", "getHighSpeed", "getIdleCurrent", "getLowSpeed", "getMode", "getPolarity", "getPosition", "getProductId", "getRunCurrent", "getStatus", "homeMotorNeg", "homeMotorPos", "initialize", "jogConstNeg", "jogConstPos", "moveToPos", "openRef", "pause", "powerOFF", "powerON", "processEvents", "rawCmd", "setAcceleration", "setDeviceId", "setDigOutput", "setHighSpeed", "setLowSpeed", "setPolarity", "setPosition", "setRunCurrent", "setIdleCurrent", "setMode", "setTimeOuts", "stopImmediately", "stopSlowly", "storeToFlashMem", "updatePanelItems", "validateDemoPos", "validatePos", "waitUntilDone", "zeroPosition"] ("actions")
                  }
                  frame "stop quick" {
                    w373 = T7[] [enum."stopImmediately", enum."processEvents"] items=["about", "clearError", "closeRef", "demo", "getAcceleration", "getActualCurrentVal", "getDeviceId", "getDeviceList", "getDigInputs", "getDigOutputs", "getDriverPowerStatus", "getFirmwareVer", "getHighSpeed", "getIdleCurrent", "getLowSpeed", "getMode", "getPolarity", "getPosition", "getProductId", "getRunCurrent", "getStatus", "homeMotorNeg", "homeMotorPos", "initialize", "jogConstNeg", "jogConstPos", "moveToPos", "openRef", "pause", "powerOFF", "powerON", "processEvents", "rawCmd", "setAcceleration", "setDeviceId", "setDigOutput", "setHighSpeed", "setLowSpeed", "setPolarity", "setPosition", "setRunCurrent", "setIdleCurrent", "setMode", "setTimeOuts", "stopImmediately", "stopSlowly", "storeToFlashMem", "updatePanelItems", "validateDemoPos", "validatePos", "waitUntilDone", "zeroPosition"] ("actions")
                  }
                  frame "stop slow" {
                    w374 = T7[] [enum."stopSlowly", enum."processEvents"] items=["about", "clearError", "closeRef", "demo", "getAcceleration", "getActualCurrentVal", "getDeviceId", "getDeviceList", "getDigInputs", "getDigOutputs", "getDriverPowerStatus", "getFirmwareVer", "getHighSpeed", "getIdleCurrent", "getLowSpeed", "getMode", "getPolarity", "getPosition", "getProductId", "getRunCurrent", "getStatus", "homeMotorNeg", "homeMotorPos", "initialize", "jogConstNeg", "jogConstPos", "moveToPos", "openRef", "pause", "powerOFF", "powerON", "processEvents", "rawCmd", "setAcceleration", "setDeviceId", "setDigOutput", "setHighSpeed", "setLowSpeed", "setPolarity", "setPosition", "setRunCurrent", "setIdleCurrent", "setMode", "setTimeOuts", "stopImmediately", "stopSlowly", "storeToFlashMem", "updatePanelItems", "validateDemoPos", "validatePos", "waitUntilDone", "zeroPosition"] ("actions")
                  }
                  frame "toggle on/off" {
                    n139 = local read "on/off"() -> (w375:bool)
                    n140 = case shown="False" w375 {
                      tunnel: [w377 w378] -> w376
                      frame True {
                        w377 = T7[] [enum."powerOFF", enum."processEvents"] items=["about", "clearError", "closeRef", "demo", "getAcceleration", "getActualCurrentVal", "getDeviceId", "getDeviceList", "getDigInputs", "getDigOutputs", "getDriverPowerStatus", "getFirmwareVer", "getHighSpeed", "getIdleCurrent", "getLowSpeed", "getMode", "getPolarity", "getPosition", "getProductId", "getRunCurrent", "getStatus", "homeMotorNeg", "homeMotorPos", "initialize", "jogConstNeg", "jogConstPos", "moveToPos", "openRef", "pause", "powerOFF", "powerON", "processEvents", "rawCmd", "setAcceleration", "setDeviceId", "setDigOutput", "setHighSpeed", "setLowSpeed", "setPolarity", "setPosition", "setRunCurrent", "setIdleCurrent", "setMode", "setTimeOuts", "stopImmediately", "stopSlowly", "storeToFlashMem", "updatePanelItems", "validateDemoPos", "validatePos", "waitUntilDone", "zeroPosition"] ("actions")
                      }
                      frame False {
                        w378 = T7[] [enum."powerON", enum."processEvents"] items=["about", "clearError", "closeRef", "demo", "getAcceleration", "getActualCurrentVal", "getDeviceId", "getDeviceList", "getDigInputs", "getDigOutputs", "getDriverPowerStatus", "getFirmwareVer", "getHighSpeed", "getIdleCurrent", "getLowSpeed", "getMode", "getPolarity", "getPosition", "getProductId", "getRunCurrent", "getStatus", "homeMotorNeg", "homeMotorPos", "initialize", "jogConstNeg", "jogConstPos", "moveToPos", "openRef", "pause", "powerOFF", "powerON", "processEvents", "rawCmd", "setAcceleration", "setDeviceId", "setDigOutput", "setHighSpeed", "setLowSpeed", "setPolarity", "setPosition", "setRunCurrent", "setIdleCurrent", "setMode", "setTimeOuts", "stopImmediately", "stopSlowly", "storeToFlashMem", "updatePanelItems", "validateDemoPos", "validatePos", "waitUntilDone", "zeroPosition"] ("actions")
                      }
                    }
                  }
                  frame Default {
                    w382 = T7[] [enum."processEvents"] items=["about", "clearError", "closeRef", "demo", "getAcceleration", "getActualCurrentVal", "getDeviceId", "getDeviceList", "getDigInputs", "getDigOutputs", "getDriverPowerStatus", "getFirmwareVer", "getHighSpeed", "getIdleCurrent", "getLowSpeed", "getMode", "getPolarity", "getPosition", "getProductId", "getRunCurrent", "getStatus", "homeMotorNeg", "homeMotorPos", "initialize", "jogConstNeg", "jogConstPos", "moveToPos", "openRef", "pause", "powerOFF", "powerON", "processEvents", "rawCmd", "setAcceleration", "setDeviceId", "setDigOutput", "setHighSpeed", "setLowSpeed", "setPolarity", "setPosition", "setRunCurrent", "setIdleCurrent", "setMode", "setTimeOuts", "stopImmediately", "stopSlowly", "storeToFlashMem", "updatePanelItems", "validateDemoPos", "validatePos", "waitUntilDone", "zeroPosition"] ("actions")
                    n141 = Format Into String(format string="Unknown Menu Item '%s'" ("message"), w379) -> (resulting string=w380:string)  [unwired: 2 in, 1 out]
                    n142 = One Button Dialog(message=w380) -> ()  [unwired: 1 in, 1 out]
                  }
                }
              }
              event "polarities": Value Change {
                w383 = T7[] [enum."setPolarity", enum."processEvents"] items=["about", "clearError", "closeRef", "demo", "getAcceleration", "getActualCurrentVal", "getDeviceId", "getDeviceList", "getDigInputs", "getDigOutputs", "getDriverPowerStatus", "getFirmwareVer", "getHighSpeed", "getIdleCurrent", "getLowSpeed", "getMode", "getPolarity", "getPosition", "getProductId", "getRunCurrent", "getStatus", "homeMotorNeg", "homeMotorPos", "initialize", "jogConstNeg", "jogConstPos", "moveToPos", "openRef", "pause", "powerOFF", "powerON", "processEvents", "rawCmd", "setAcceleration", "setDeviceId", "setDigOutput", "setHighSpeed", "setLowSpeed", "setPolarity", "setPosition", "setRunCurrent", "setIdleCurrent", "setMode", "setTimeOuts", "stopImmediately", "stopSlowly", "storeToFlashMem", "updatePanelItems", "validateDemoPos", "validatePos", "waitUntilDone", "zeroPosition"] ("actions")
                n143 = event-data() -> ()  [unwired: 1 in, 6 out]
              }
              event "help": Value Change {
                w387 = T7[] [enum."processEvents"] items=["about", "clearError", "closeRef", "demo", "getAcceleration", "getActualCurrentVal", "getDeviceId", "getDeviceList", "getDigInputs", "getDigOutputs", "getDriverPowerStatus", "getFirmwareVer", "getHighSpeed", "getIdleCurrent", "getLowSpeed", "getMode", "getPolarity", "getPosition", "getProductId", "getRunCurrent", "getStatus", "homeMotorNeg", "homeMotorPos", "initialize", "jogConstNeg", "jogConstPos", "moveToPos", "openRef", "pause", "powerOFF", "powerON", "processEvents", "rawCmd", "setAcceleration", "setDeviceId", "setDigOutput", "setHighSpeed", "setLowSpeed", "setPolarity", "setPosition", "setRunCurrent", "setIdleCurrent", "setMode", "setTimeOuts", "stopImmediately", "stopSlowly", "storeToFlashMem", "updatePanelItems", "validateDemoPos", "validatePos", "waitUntilDone", "zeroPosition"] ("actions")
                n144 = event-data() -> ()  [unwired: 1 in, 6 out]
                n145 = fn#1354() -> (1:w386:bool)  [unwired: 1 out]
                n146 = Not(x=w386) -> (.not. x?=w385:bool)
                n147 = Control Help Window(1:w385) -> ()  [unwired: 1 in]
              }
              event "dig_outs", "polarities.Digital Output": Value Change {
                w389 = T7[] [enum."setDigOutput", enum."processEvents"] items=["about", "clearError", "closeRef", "demo", "getAcceleration", "getActualCurrentVal", "getDeviceId", "getDeviceList", "getDigInputs", "getDigOutputs", "getDriverPowerStatus", "getFirmwareVer", "getHighSpeed", "getIdleCurrent", "getLowSpeed", "getMode", "getPolarity", "getPosition", "getProductId", "getRunCurrent", "getStatus", "homeMotorNeg", "homeMotorPos", "initialize", "jogConstNeg", "jogConstPos", "moveToPos", "openRef", "pause", "powerOFF", "powerON", "processEvents", "rawCmd", "setAcceleration", "setDeviceId", "setDigOutput", "setHighSpeed", "setLowSpeed", "setPolarity", "setPosition", "setRunCurrent", "setIdleCurrent", "setMode", "setTimeOuts", "stopImmediately", "stopSlowly", "storeToFlashMem", "updatePanelItems", "validateDemoPos", "validatePos", "waitUntilDone", "zeroPosition"] ("actions")
                n148 = event-data() -> ()  [unwired: 1 in, 6 out]
              }
              event "move_mode": Value Change {
                w391 = T7[] [enum."setMode", enum."processEvents"] items=["about", "clearError", "closeRef", "demo", "getAcceleration", "getActualCurrentVal", "getDeviceId", "getDeviceList", "getDigInputs", "getDigOutputs", "getDriverPowerStatus", "getFirmwareVer", "getHighSpeed", "getIdleCurrent", "getLowSpeed", "getMode", "getPolarity", "getPosition", "getProductId", "getRunCurrent", "getStatus", "homeMotorNeg", "homeMotorPos", "initialize", "jogConstNeg", "jogConstPos", "moveToPos", "openRef", "pause", "powerOFF", "powerON", "processEvents", "rawCmd", "setAcceleration", "setDeviceId", "setDigOutput", "setHighSpeed", "setLowSpeed", "setPolarity", "setPosition", "setRunCurrent", "setIdleCurrent", "setMode", "setTimeOuts", "stopImmediately", "stopSlowly", "storeToFlashMem", "updatePanelItems", "validateDemoPos", "validatePos", "waitUntilDone", "zeroPosition"] ("actions")
                n149 = event-data() -> ()  [unwired: 1 in, 6 out]
              }
            }
          }
          frame "rawCmd" {
            # "avoid shutting\ndown the app\nin the event\nincorrectly \nformatted commands\nare entered."
            n150 = call "send_receive_command.vi"("reference (in)"=w395, "command (raw)"="raw_cmd", "error in (no error)"=w400) -> ("reference (dup)"=w394:i32, "read_string"=→"response":string)  [unwired: 8 in, 3 out]
          }
          frame "setAcceleration" {
            n151 = Number To Decimal String(number="accel") -> (decimal integer string=w403:string)  [unwired: 1 in]
            n152 = Build Array(w403) -> (w402:string[])
            n153 = call "send_receive_command.vi"("reference (in)"=w406, "command"=commands."set acceleration" ("commands"), "params (opt)"=w402, "error in (no error)"=w408) -> ("reference (dup)"=w405:i32, "error out"=w407:errorcluster)  [unwired: 7 in, 3 out]
            n154 = Build Array (concatenate)(utility_actions."getAcceleration" ("Enum"), w411) -> (w410:T7[])
          }
          frame "setDeviceId" {
            w416 = FALSE  # echo errors? (T)
            n155 = Build Array("new_id") -> (w418:string[])
            n156 = call "send_receive_command.vi"("reference (in)"=w421, "command"=commands."set device id" ("commands"), "params (opt)"=w418, "error in (no error)"=w422, "echo errors? (T)"=w416) -> ("reference (dup)"=w420:i32, "error out"=w415:errorcluster)  [unwired: 6 in, 3 out]
            n157 = case shown="No Error" w415 {
              selector: w415 -> [w427 _]
              tunnel: [w427 errorcluster {"status"=FALSE, "code"=0, "source"=""} ("error out")] -> w414
              tunnel: [w426 w428] -> w413
              frame No Error {
                w426 = T7[] [enum."getDeviceId", enum."storeToFlashMem"] items=["about", "clearError", "closeRef", "demo", "getAcceleration", "getActualCurrentVal", "getDeviceId", "getDeviceList", "getDigInputs", "getDigOutputs", "getDriverPowerStatus", "getFirmwareVer", "getHighSpeed", "getIdleCurrent", "getLowSpeed", "getMode", "getPolarity", "getPosition", "getProductId", "getRunCurrent", "getStatus", "homeMotorNeg", "homeMotorPos", "initialize", "jogConstNeg", "jogConstPos", "moveToPos", "openRef", "pause", "powerOFF", "powerON", "processEvents", "rawCmd", "setAcceleration", "setDeviceId", "setDigOutput", "setHighSpeed", "setLowSpeed", "setPolarity", "setPosition", "setRunCurrent", "setIdleCurrent", "setMode", "setTimeOuts", "stopImmediately", "stopSlowly", "storeToFlashMem", "updatePanelItems", "validateDemoPos", "validatePos", "waitUntilDone", "zeroPosition"]
              }
              frame Error {
                w428 = T7[] [] items=["about", "clearError", "closeRef", "demo", "getAcceleration", "getActualCurrentVal", "getDeviceId", "getDeviceList", "getDigInputs", "getDigOutputs", "getDriverPowerStatus", "getFirmwareVer", "getHighSpeed", "getIdleCurrent", "getLowSpeed", "getMode", "getPolarity", "getPosition", "getProductId", "getRunCurrent", "getStatus", "homeMotorNeg", "homeMotorPos", "initialize", "jogConstNeg", "jogConstPos", "moveToPos", "openRef", "pause", "powerOFF", "powerON", "processEvents", "rawCmd", "setAcceleration", "setDeviceId", "setDigOutput", "setHighSpeed", "setLowSpeed", "setPolarity", "setPosition", "setRunCurrent", "setIdleCurrent", "setMode", "setTimeOuts", "stopImmediately", "stopSlowly", "storeToFlashMem", "updatePanelItems", "validateDemoPos", "validatePos", "waitUntilDone", "zeroPosition"]
                n158 = One Button Dialog(message="An error was detected while\nattempting to change the \nDevice ID.  Please check the\nformatting of the ID and \ntry again.") -> ()  [unwired: 1 in, 1 out]
              }
            }
            n159 = Build Array (concatenate)(w413, w424) -> (w423:T7[])
          }
          frame "setDigOutput" {
            n160 = Unbundle By Name("dig_outs") -> ("Digital Output 2"=w432:bool, "Digital Output 1"=w431:bool)
            n161 = call "set_digital_output_value.vi"("reference (in)"=w438, "digital_output_ch"=digital_output_items."DIG_OUT_1", "dig_out_value"=w431, "error in (no error)"=w440) -> ("reference (dup)"=w435:i32, "error out"=w439:errorcluster)  [unwired: 13 in, 1 out]
            n162 = call "set_digital_output_value.vi"("reference (in)"=w435, "digital_output_ch"=digital_output_items."DIG_OUT_2", "dig_out_value"=w432) -> ("reference (dup)"=w434:i32)  [unwired: 14 in, 2 out]
            n163 = Build Array (concatenate)(utility_actions."getDigOutputs" ("Enum"), w443) -> (w442:T7[])
          }
          frame "setHighSpeed" {
            n164 = Number To Decimal String(number="high_speed") -> (decimal integer string=w448:string)  [unwired: 1 in]
            n165 = Build Array(w448) -> (w447:string[])
            n166 = call "send_receive_command.vi"("reference (in)"=w451, "command"=commands."set high speed" ("commands"), "params (opt)"=w447, "error in (no error)"=w453) -> ("reference (dup)"=w450:i32, "error out"=w452:errorcluster)  [unwired: 7 in, 3 out]
            n167 = Build Array (concatenate)(utility_actions."getHighSpeed" ("Enum"), w455) -> (w454:T7[])
          }
          frame "setLowSpeed" {
            n168 = Number To Decimal String(number="low_speed") -> (decimal integer string=w460:string)  [unwired: 1 in]
            n169 = Build Array(w460) -> (w459:string[])
            n170 = call "send_receive_command.vi"("reference (in)"=w463, "command"=commands."set low speed" ("commands"), "params (opt)"=w459, "error in (no error)"=w465) -> ("reference (dup)"=w462:i32, "error out"=w464:errorcluster)  [unwired: 7 in, 3 out]
            n171 = Build Array (concatenate)(utility_actions."getLowSpeed" ("Enum"), w467) -> (w466:T7[])
          }
          frame "setPolarity" {
            n172 = Cluster To Array(cluster="polarities") -> (array=w471:bool[])
            n173 = for {
              tunnel: w471 -> [w480] mode=indexing
              tunnel: T11[] [{"item"=enum."DIRECTION", "status"=FALSE}, {"item"=enum."LIMIT", "status"=FALSE}, {"item"=enum."HOME", "status"=FALSE}, {"item"=enum."DIG_OUT", "status"=FALSE}, {"item"=enum."DIG_IN", "status"=FALSE}, {"item"=enum."ENABLE_OUT", "status"=FALSE}, {"item"=enum."JUMP_ERR", "status"=FALSE}] ("polarity_items") -> [w481] mode=indexing
              tunnel: [w479] -> w469 mode=indexing
              n174 = Bundle By Name(cluster=w481, "status"=w480) -> (w479:T11)
            }
            n175 = call "set_polarity_values.vi"("reference (in)"=w474, "polarity_items"=w469, "error in (no error)"=w476) -> ("reference (dup)"=w473:i32, "error out"=w475:errorcluster)  [unwired: 14 in, 1 out]
          }
          frame "setPosition" {
            n176 = Number To Decimal String(number="position_val_desired") -> (decimal integer string=w485:string)  [unwired: 1 in]
            n177 = Build Array(w485) -> (w484:string[])
            n178 = call "send_receive_command.vi"("reference (in)"=w488, "command"=commands."set position" ("commands"), "params (opt)"=w484, "error in (no error)"=w490) -> ("reference (dup)"=w487:i32, "error out"=w489:errorcluster)  [unwired: 7 in, 3 out]
            n179 = Build Array (concatenate)(utility_actions."getPosition" ("Enum"), w492) -> (w491:T7[])
          }
          frame "setMode" {
            n180 = case shown="\"Abs:\"" "move_mode" {
              tunnel: [commands."set move mode increment" ("commands") commands."set move mode absolute" ("commands")] -> w494
              frame "Inc:" {
              }
              frame "Abs:" {
              }
            }
            n181 = call "send_receive_command.vi"("reference (in)"=w498, "command"=w494, "error in (no error)"=w500) -> ("reference (dup)"=w497:i32, "error out"=w499:errorcluster)  [unwired: 8 in, 3 out]
            n182 = Build Array (concatenate)(utility_actions."getMode" ("Enum"), w502) -> (w501:T7[])
          }
          frame "setRunCurrent" {
            n183 = Number To Decimal String(number="running_amp") -> (decimal integer string=w509:string)  [unwired: 1 in]
            n184 = Build Array(w509) -> (w508:string[])
            n185 = call "send_receive_command.vi"("reference (in)"=w512, "command"=commands."set run current" ("commands"), "params (opt)"=w508, "error in (no error)"=w514) -> ("reference (dup)"=w511:i32, "error out"=w513:errorcluster)  [unwired: 7 in, 3 out]
            n186 = Build Array (concatenate)(utility_actions."getRunCurrent" ("Enum"), w516) -> (w515:T7[])
          }
          frame "setIdleCurrent" {
            n187 = Number To Decimal String(number="idle_amp") -> (decimal integer string=w521:string)  [unwired: 1 in]
            n188 = Build Array(w521) -> (w520:string[])
            n189 = call "send_receive_command.vi"("reference (in)"=w524, "command"=commands."set idle current" ("commands"), "params (opt)"=w520, "error in (no error)"=w526) -> ("reference (dup)"=w523:i32, "error out"=w525:errorcluster)  [unwired: 7 in, 3 out]
            n190 = Build Array (concatenate)(utility_actions."getIdleCurrent" ("Enum"), w528) -> (w527:T7[])
          }
          frame "setTimeOuts" {
            w531 = 1000  # write_timeout (ms)
            w532 = 1000  # read_timeout (ms)
            n191 = call "set_timeouts.vi"("read_timeout (ms); def=1000"=w532, "write_timeout (ms); def=1000"=w531, "error in (no error)"=w534) -> ("error out"=w533:errorcluster)  [unwired: 12 in]
          }
          frame "stopImmediately" {
            w537 = u8 0 ("Disabled")
            n192 = call "send_receive_command.vi"("reference (in)"=w540, "command"=commands."stop immediate" ("commands"), "error in (no error)"=w542) -> ("reference (dup)"=w539:i32, "error out"=w541:errorcluster)  [unwired: 8 in, 3 out]
            n193 = property on="home_neg" class="Bool"("Disabled"=w537) -> ()  [unwired: 2 in, 2 out]
            n194 = property on="home_pos" class="Bool"("Disabled"=w537) -> ()  [unwired: 2 in, 2 out]
            n195 = property on="move_to" class="Bool"("Disabled"=w537) -> ()  [unwired: 2 in, 2 out]
            n196 = property on="jog_pos" class="Bool"("Disabled"=w537) -> ()  [unwired: 2 in, 2 out]
            n197 = property on="jog_neg" class="Bool"("Disabled"=w537) -> ()  [unwired: 2 in, 2 out]
          }
          frame "stopSlowly" {
            w545 = u8 0 ("Disabled")
            n198 = call "send_receive_command.vi"("reference (in)"=w548, "command"=commands."stop slow" ("commands"), "error in (no error)"=w550) -> ("reference (dup)"=w547:i32, "error out"=w549:errorcluster)  [unwired: 8 in, 3 out]
            n199 = property on="home_neg" class="Bool"("Disabled"=w545) -> ()  [unwired: 2 in, 2 out]
            n200 = property on="home_pos" class="Bool"("Disabled"=w545) -> ()  [unwired: 2 in, 2 out]
            n201 = property on="move_to" class="Bool"("Disabled"=w545) -> ()  [unwired: 2 in, 2 out]
            n202 = property on="jog_pos" class="Bool"("Disabled"=w545) -> ()  [unwired: 2 in, 2 out]
            n203 = property on="jog_neg" class="Bool"("Disabled"=w545) -> ()  [unwired: 2 in, 2 out]
          }
          frame "updatePanelItems" {
            w555 = T7[] [] items=["about", "clearError", "closeRef", "demo", "getAcceleration", "getActualCurrentVal", "getDeviceId", "getDeviceList", "getDigInputs", "getDigOutputs", "getDriverPowerStatus", "getFirmwareVer", "getHighSpeed", "getIdleCurrent", "getLowSpeed", "getMode", "getPolarity", "getPosition", "getProductId", "getRunCurrent", "getStatus", "homeMotorNeg", "homeMotorPos", "initialize", "jogConstNeg", "jogConstPos", "moveToPos", "openRef", "pause", "powerOFF", "powerON", "processEvents", "rawCmd", "setAcceleration", "setDeviceId", "setDigOutput", "setHighSpeed", "setLowSpeed", "setPolarity", "setPosition", "setRunCurrent", "setIdleCurrent", "setMode", "setTimeOuts", "stopImmediately", "stopSlowly", "storeToFlashMem", "updatePanelItems", "validateDemoPos", "validatePos", "waitUntilDone", "zeroPosition"] ("actions")
            n204 = Build Array (concatenate)(w555, w556) -> (w554:T7[])
          }
          frame "validateDemoPos" {
            w569 = 262143
            n205 = local read "position_val_actual"() -> (w577:i32)
            n206 = Add(x=w577, y=w569) -> (x+y=w576:i32)
            n207 = Subtract(x=w577, y=w569) -> (x-y=w575:i32)
            n208 = Add(x="pos_1", y=w569) -> (x+y=w573:i32)
            n209 = Subtract(x="pos_1", y=w569) -> (x-y=w574:i32)
            n210 = Add(x="pos_2", y=w569) -> (x+y=w572:i32)
            n211 = Subtract(x="pos_2", y=w569) -> (x-y=w571:i32)
            n212 = In Range and Coerce(upper limit=w576, x="pos_1", lower limit=w575) -> (In Range?=w566:bool)  [unwired: 1 out]
            n213 = In Range and Coerce(upper limit=w573, x="pos_2", lower limit=w574) -> (In Range?=w567:bool)  [unwired: 1 out]
            n214 = In Range and Coerce(upper limit=w572, x="pos_3", lower limit=w571) -> (In Range?=w565:bool)  [unwired: 1 out]
            n215 = Compound Arithmetic op=AND(w566, w567, w565) -> (w563:bool)
            n216 = case shown="False" w563 {
              tunnel: w564 -> [_ w583]
              tunnel: w561 -> [w582 w584]
              tunnel: [w582 w584] -> w562
              tunnel: [w581 w583] -> w560
              frame False {
                w581 = T7[] [enum."processEvents"] items=["about", "clearError", "closeRef", "demo", "getAcceleration", "getActualCurrentVal", "getDeviceId", "getDeviceList", "getDigInputs", "getDigOutputs", "getDriverPowerStatus", "getFirmwareVer", "getHighSpeed", "getIdleCurrent", "getLowSpeed", "getMode", "getPolarity", "getPosition", "getProductId", "getRunCurrent", "getStatus", "homeMotorNeg", "homeMotorPos", "initialize", "jogConstNeg", "jogConstPos", "moveToPos", "openRef", "pause", "powerOFF", "powerON", "processEvents", "rawCmd", "setAcceleration", "setDeviceId", "setDigOutput", "setHighSpeed", "setLowSpeed", "setPolarity", "setPosition", "setRunCurrent", "setIdleCurrent", "setMode", "setTimeOuts", "stopImmediately", "stopSlowly", "storeToFlashMem", "updatePanelItems", "validateDemoPos", "validatePos", "waitUntilDone", "zeroPosition"] ("actions")
                n217 = One Button Dialog(message="all position values must \nfall within +/- 262143\nticks of the previous \nposition.  Please make \nthe necessary corrections\nand try again.") -> ()  [unwired: 1 in, 1 out]
              }
              frame True {
              }
            }
          }
          frame "validatePos" {
            w591 = 262143
            n218 = local read "position_val_actual"() -> (w594:i32)
            n219 = Add(x=w594, y=w591) -> (x+y=w593:i32)
            n220 = Subtract(x=w594, y=w591) -> (x-y=w592:i32)
            n221 = In Range and Coerce(upper limit=w593, x="jog_to_pos", lower limit=w592) -> (In Range?=w585:bool)  [unwired: 1 out]
            n222 = case shown="False" w585 {
              tunnel: w590 -> [_ w600]
              tunnel: w588 -> [w599 w601]
              tunnel: [w599 w601] -> w589
              tunnel: [w598 w600] -> w587
              frame False {
                w598 = T7[] [enum."processEvents"] items=["about", "clearError", "closeRef", "demo", "getAcceleration", "getActualCurrentVal", "getDeviceId", "getDeviceList", "getDigInputs", "getDigOutputs", "getDriverPowerStatus", "getFirmwareVer", "getHighSpeed", "getIdleCurrent", "getLowSpeed", "getMode", "getPolarity", "getPosition", "getProductId", "getRunCurrent", "getStatus", "homeMotorNeg", "homeMotorPos", "initialize", "jogConstNeg", "jogConstPos", "moveToPos", "openRef", "pause", "powerOFF", "powerON", "processEvents", "rawCmd", "setAcceleration", "setDeviceId", "setDigOutput", "setHighSpeed", "setLowSpeed", "setPolarity", "setPosition", "setRunCurrent", "setIdleCurrent", "setMode", "setTimeOuts", "stopImmediately", "stopSlowly", "storeToFlashMem", "updatePanelItems", "validateDemoPos", "validatePos", "waitUntilDone", "zeroPosition"] ("actions")
                n223 = One Button Dialog(message="all position values must \nfall within +/- 262143\nticks of the current \nposition.  Please make \nthe necessary corrections\nand try again.") -> ()  [unwired: 1 in, 1 out]
              }
              frame True {
              }
            }
          }
          frame "zeroPosition" {
            n224 = Number To Decimal String(number=0) -> (decimal integer string=w604:string)  [unwired: 1 in]
            n225 = Build Array(w604) -> (w606:string[])
            n226 = call "send_receive_command.vi"("reference (in)"=w608, "command"=commands."set position" ("commands"), "params (opt)"=w606, "error in (no error)"=w610) -> ("reference (dup)"=w607:i32, "error out"=w609:errorcluster)  [unwired: 7 in, 3 out]
            n227 = Build Array (concatenate)(utility_actions."getPosition" ("Enum"), w612) -> (w611:T7[])
          }
        }
        n228 = Array Size(array=w29) -> (size(s)=w28:i32)
        n229 = Unbundle By Name(w24) -> ("status"=w26:bool)
        n230 = Equal To 0?(x=w28) -> (x = 0?=w27:bool)
        n231 = Or(x=w27, y=w26) -> (x .or. y?=w25:bool)
      }
      n232 = case shown="Error" w7 {
        selector: w7 -> [w13 w16]
        tunnel: w6 -> [_ w19]
        tunnel: [w13 w18] -> w4
        frame No Error {
        }
        frame Error {
          # "In case of unexpected\nerrors, close connection"
          n233 = Unbundle By Name(w16) -> ("source"=w15:string)
          n234 = Build Array(w15) -> (w14:string[])
          n235 = call "errors.vi"("errors"=errors_actions."unknown", "supp_text"=w14) -> ()  [unwired: 13 in, 1 out]
          n236 = call "close_connection.vi"("reference"=w19) -> ("error out"=w18:errorcluster)  [unwired: 14 in]
        }
      }
      n237 = flat-sequence {
        tunnel: w4 -> [w10]
        tunnel: [w10] -> w3
        frame #0 {
          n238 = Current VI's Path() -> (path=w12:path)
          n239 = call "get_exe_home_path.vi"("home_path"=w12) -> ("running in an executable?"=w11:bool)  [unwired: 6 in, 1 out]
          n240 = Quit LabVIEW(quit? (T)=w11) -> ()
        }
      }
    }
    frame Error {
    }
  }
  "error out" <- w1
